vi "MoD Main-Optimize - Simulate.vi"() -> ()   [LabVIEW 2015]
uses:
  <vilib>/ni845x/ni845x.llb/ni845xControl.ctl
  <vilib>/addons/control/pid/pid.llb/PID Control Input Filter (DBL).vi
  <vilib>/addons/control/pid/autopid.llb/PID Online Autotuning (Relay Feedback).vi
  <vilib>/addons/control/pid/NI_PID_autopid.lvlib
  <vilib>/addons/control/pid/NI_PID_pid.lvlib
  <vilib>/DAQmx/read.llb/DAQmx Read (Analog 1D DBL NChan 1Samp).vi
  <vilib>/DAQmx/create/channels.llb/DAQmx Create Channel (AI-Voltage-Basic).vi
panel:
  out "stop_xl_write":bool=TRUE
  out "Num_exp_till_pause":i32
  out "Syringe_pump?":bool=TRUE
  out "System Error":bool=TRUE
  out "error out":errorcluster
  out "MS task":refnum<k21>
  out "MS Array":dbl[](array[numeric]) format="%0.2f"
  out "Pump setpoint(ul/min) 6":dbl format="%#_13g"
  out "Pump setpoint(ul/min) 5":dbl format="%#_13g"
  out "Pump setpoint(ul/min) 4":dbl format="%#_13g"
  out "Pump setpoint(ul/min) 3":dbl format="%#_13g"
  out "Pump setpoint(ul/min) 2":dbl format="%#_13g"
  out "Pump setpoint(ul/min) 1":dbl format="%#_13g"
  out "Volume (ul) 5":dbl format="%#_13g"
  out "Volume (ul) 4":dbl format="%#_13g"
  out "Volume (ul) 3":dbl format="%#_13g"
  out "Volume (ul) 2":dbl format="%#_13g"
  out "Volume (ul) 1":dbl format="%#_13g"
  in  "tau 5":dbl format="%#_13g"
  out "tau 4":dbl format="%#_13g"
  out "tau 3":dbl format="%#_13g"
  out "tau 2":dbl format="%#_13g"
  out "tau 1":dbl format="%#_13g"
  out "Reactor Length":dbl format="%#_13g"
  out "Flowrate Sensor 2":dbl format="%#_13g"
  out "Flowrate Sensor 1":dbl format="%#_13g"
  out "Pressure 2":dbl format="%#_13g"
  out "Pressure 1":dbl format="%#_13g"
  out "Temperature Control 5":bool=TRUE
  out "Temperature Control 4":bool=TRUE
  out "Temperature Control 3":bool=TRUE
  out "Temperature Control 2":bool=TRUE
  out "Temperature Control 1":bool=TRUE
  out "Temperature SP 5":dbl format="%#_g'C"
  out "Temperature SP 4":dbl format="%#_g'C"
  out "Temperature SP 3":dbl format="%#_g'C"
  out "Temperature SP 2":dbl format="%#_g'C"
  out "Temperature SP 1":dbl format="%#_g'C"
  in  "Bay Temperature 5":dbl
  in  "SSR Duration 5":dbl
  in  "SSR Duration 4":dbl
  in  "SSR Duration 3":dbl
  in  "SSR Duration 2":dbl
  in  "SSR Duration 1":dbl
  in  "Total Product Amount":dbl=1.0 format="%#_gml"
  out "Setup Error":bool=TRUE
  out "Error Message":string
  out "ID CTR":i32
  in  "Tab Control 2":enum32{"Faults", "Devices"}(tab)=enum."Devices"
  out "Fault Cluster":T1
  in  "COMM Port:: Harvard Syringe Pump":refnum<visa-resource-name>
  in  "Sample Valve COMM::Port":refnum<visa-resource-name>
  in  "Arduino COMM Port":refnum<visa-resource-name>
  in  "COMM Port :: Milligat Pumps":refnum<visa-resource-name>
  in  "IR Sensor Device":T2
  in  "MS Analog Channel":tag
  in  "Tab Control":T3(tab)
  in  "System decide help Button":bool
  in  "Reaction Scheme Confirm":bool
  in  "Synthesis Route Array":string[](array[string])=["Aldehyde", "Amine", "BoroHydride", "Aqueous Salt", "", ""]
  in  "Manual/Automated":bool
  in  "Save Button":bool
  in  "Open Button":bool
  in  "New rxn scheme button":bool
  in  "System decide help Button 2":bool
  out "Setup Confirm":bool=TRUE
  in  "BAY 1":u16(ring) items=["                 Bypass", "             Hot Reactor", "               Separator"]
  in  "BAY 5":u16(ring)=2 items=["                     Bypass", "                Hot Reactor", "                 Separator"]
  in  "BAY 4":u16(ring) items=["                     Bypass", "                Hot Reactor", "                  Separator"]
  in  "BAY 3":u16(ring)=1 items=["                     Bypass", "                 Hot Reactor", "                  Separator"]
  in  "BAY 2":u16(ring)=1 items=["                     Bypass", "                Hot Reactor", "                  Separator"]
  out "Paramter Confirm":bool=TRUE
  in  "System Parameters Help Button":bool
  in  "System Parameters Confirm Button":bool
  in  "Bay Parameters":T4={"Pump 1 Reagent Concentration"=2.0, "Pump 2 Reagent Concentration"=2.0, "Pump 3 Reagent Concentration"=2.0, "Pump 4 Reagent Concentration"=2.0, "Pump 5 Reagent Concentration"=2.0, "Bay 1 Parameters"={"Pump 1 Flowrate"=0.0, "optimize_temp"=TRUE, "optimize_tau"=TRUE, "Run at set flowrate"=FALSE, "Pump 2 Flowrate"=0.0, "Temperature Params"=[0.0, 25.0, 100.0], "Resisdence time params"=[0.0, 0.5, 15.0], "Resisdence time params 2"=[0.0, 0.5, 15.0]}, "Bay 2 Parameters"={"Pump 3 Flowrate"=0.0, "optimize_temp"=TRUE, "optimize_tau"=TRUE, "Run at set flowrate"=FALSE, "Temperature Params"=[0.0, 25.0, 100.0], "Resisdence time params"=[0.0, 0.5, 15.0], "pump_at_ratio"=FALSE, "pump_num_ratio"=0.0}, "Bay 3 Parameters"={"Pump 4 Flowrate"=0.0, "optimize_temp"=FALSE, "optimize_tau"=FALSE, "Run at set flowrate"=FALSE, "Temperature Params"=[0.0, 0.0, 0.0], "Resisdence time params"=[0.0, 0.0, 0.0], "pump_at_ratio"=TRUE, "pump_num_ratio"=1.5}, "Bay 4 Parameters"={"Pump 5 Flowrate"=0.0, "Run at set flowrate"=FALSE, "optimize_temp"=FALSE, "optimize_tau"=FALSE, "Resisdence time params"=[0.0, 0.0, 0.0], "Temperature Params"=[0.0, 0.0, 0.0], "pump_at_ratio"=FALSE, "pump_num_ratio"=0.0}, "Bay 5 Parameters"={"Pump 6 Flowrate"=0.0, "Run at set flowrate"=FALSE, "optimize_temp"=FALSE, "optimize_tau"=FALSE, "Resisdence time params"=[0.0, 0.0, 0.0], "Temperature Params"=[0.0, 0.0, 0.0], "pump_at_ratio"=FALSE, "pump_num_ratio"=0.0}, "Bay 1 Flow Rate Ratio \n(Pump 1: Pump 2)"=1.0, "tube_id(in)"=[enum.".03", enum.".03", enum.".03", enum.".03", enum.".03"], "xml_filename"="temp_xml", "Excel File Name"="C:\\Users\\HPLC\\Dropbox (MIT)\\MoD Files\\Data\\HWE Results\\HWE Optimization HPLC - 04112017 sim", "HPLC File Name"="C:\\Chem32\\1\\Data\\MOD", "Matlab File"="C:\\Users\\HPLC\\Dropbox (MIT)\\MoD Files\\Data\\04112017", "Syringe for Pump 2?"=TRUE, "Num_conditons_per_wait"=0.0, "Continue from previous optimization?"=FALSE, "Pump 6 Reagent Concentration"=2.0} {"Pump 6 Reagent Concentration" format="%#_6gM"; "Bay 5 Parameters"."Temperature Params" format="%#_g'C"; "Bay 4 Parameters"."Temperature Params" format="%#_g'C"; "Bay 3 Parameters"."Temperature Params" format="%#_g'C"; "Bay 2 Parameters"."Temperature Params" format="%#_g'C"; "Bay 1 Parameters"."Temperature Params" format="%#_g'C"; "Pump 5 Reagent Concentration" format="%#_6gM"; "Pump 4 Reagent Concentration" format="%#_6gM"; "Pump 3 Reagent Concentration" format="%#_6gM"; "Pump 2 Reagent Concentration" format="%#_6gM"; "Pump 1 Reagent Concentration" format="%#_6gM"}
  out "System Confirm Not Clicked":string
  in  "Debug_run_button":bool
  in  "Pump 1":bool
  in  "Flowrate 1":dbl=200.0
  in  "Pump 4":bool
  in  "Flowrate 4":dbl=200.0
  in  "Pump 5":bool
  in  "Flowrate 5":dbl=200.0
  in  "Pump 2":bool
  in  "Flowrate 2":dbl=200.0
  in  "Pump 3":bool
  in  "Flowrate 3":dbl=200.0
  in  "Pump 6":bool
  in  "Flowrate 6":dbl=200.0
  in  "Bay Heating 1":bool
  in  "Bay Heating 2":bool
  in  "Bay Heating 3":bool
  in  "Bay Heating 4":bool
  in  "Bay Heating 5":bool
  out "HPLC Analysis":bool
  out "Equlibrating Temperature":bool
  out "Flushing System":bool
  out "Calculate condition":bool
  out "System Flush Wait Time":u8(slide) scale=0.0..2150.711842843066
  out "Temperature 5":dbl format="%#_g'C"
  out "Temperature 4":dbl format="%#_g'C"
  out "Temperature 3":dbl format="%#_g'C"
  out "Temperature 2":dbl format="%#_g'C"
  out "Temperature 1":dbl format="%#_g'C"
  out "Flowrate Chart":T5(graph)
  out "Bay 5":u16(ring) items=["                     Bypass", "                   Reactor1", "               Separator"]
  out "Bay 4":u16(ring) items=["                     Bypass", "                   Reactor1", "               Separator"]
  out "Bay 3":u16(ring) items=["                     Bypass", "                   Reactor1", "               Separator"]
  out "Bay 2":u16(ring) items=["                     Bypass", "                   Reactor1", "               Separator"]
  out "Bay 1":u16(ring) items=["                     Bypass", "                   Reactor1", "               Separator"]
  out "Teperature Chart":T5(graph)
  out "Pump Setpoints Chart":T5(graph)
  out "Pressure Chart":T5(graph)
  out "MS Signals Chart":dbl[][](graph)
  out "Optimization_loop_index":i32
  out "curr_wait_time(min)":dbl
  out "total_flush_time(min)":dbl
  out "Temp SS? 5":bool=TRUE
  out "Temp SS? 4":bool=TRUE
  out "Temp SS? 3":bool=TRUE
  out "Temp SS? 2":bool=TRUE
  out "Temp SS? 1":bool=TRUE
  out "System Flushed?":bool
  out "stop_button clicked":bool
  out "Total System Resisdence Time(min)":dbl
  out "Stop":bool=TRUE
  in  "Run_Stop_cluster":T6
  # "Molecules on Demand"
  # "Synthesis Route"
  # "Reagent List"
  # "1"
  # "2"
  # "1"
  # "3"
  # "2"
  # "4"
  # "3"
  # "5"
  # "4"
  # "6"
  # "5"
  # "Product"
  # "6"
  # "Have system decide based on synthesis route"
  # "Manually enter bay configuration"
  # "System Schematic"
  # "Optimization Parameters"
  # "Bay"
  # "Tube ID (in)"
  # "1."
  # "2."
  # "3."
  # "4."
  # "5."
  # "Pause After Every"
  # "Experiments"
  # "Reporting"
  # "XML Output File Name"
  # "Excel Output File Name"
  # "HPLC File Path"
  # "MATLAB File Path"
  # "Temperature"
  # "Residence time(min)"
  # "Setpoint"
  # "Lower Bound"
  # "Upper Bound"
  # "Optimize?"
  # "-or-"
  # "Run at"
  # "times incoming flow"
  # "Temperature"
  # "Residence time(min)"
  # "Setpoint"
  # "Lower Bound"
  # "Upper Bound"
  # "Optimize?"
  # "-or-"
  # "Run at"
  # "times incoming flow"
  # "Temperature"
  # "Residence time(min)"
  # "Setpoint"
  # "Lower Bound"
  # "Upper Bound"
  # "Optimize?"
  # "-or-"
  # "Run at"
  # "times incoming flow"
  # "Temperature"
  # "Residence time(min)"
  # "Setpoint"
  # "Lower Bound"
  # "Upper Bound"
  # "Optimize?"
  # "-or-"
  # "Run at"
  # "times incoming flow"
  # "Temperature"
  # "Residence time(min)"
  # "Setpoint"
  # "Lower Bound"
  # "Upper Bound"
  # "Optimize?"
  # "Use this page to manually test the different functions of the system during standby mode"
  # "Pumps"
  # "Bay Heating"
  # "Temperature('C)"
  # "Pressure (psi)"
  # "Flowrate (ul/min)"
  # "Pump Flowrate Setpoints(ul/min)"
  # "MS Output Voltage"
  # "Experimental Steps"
  # "Calculated new conditions"
  # "Flushed System"
  # "Analyzed HPLC"
  # "Equilibrated Temperature"
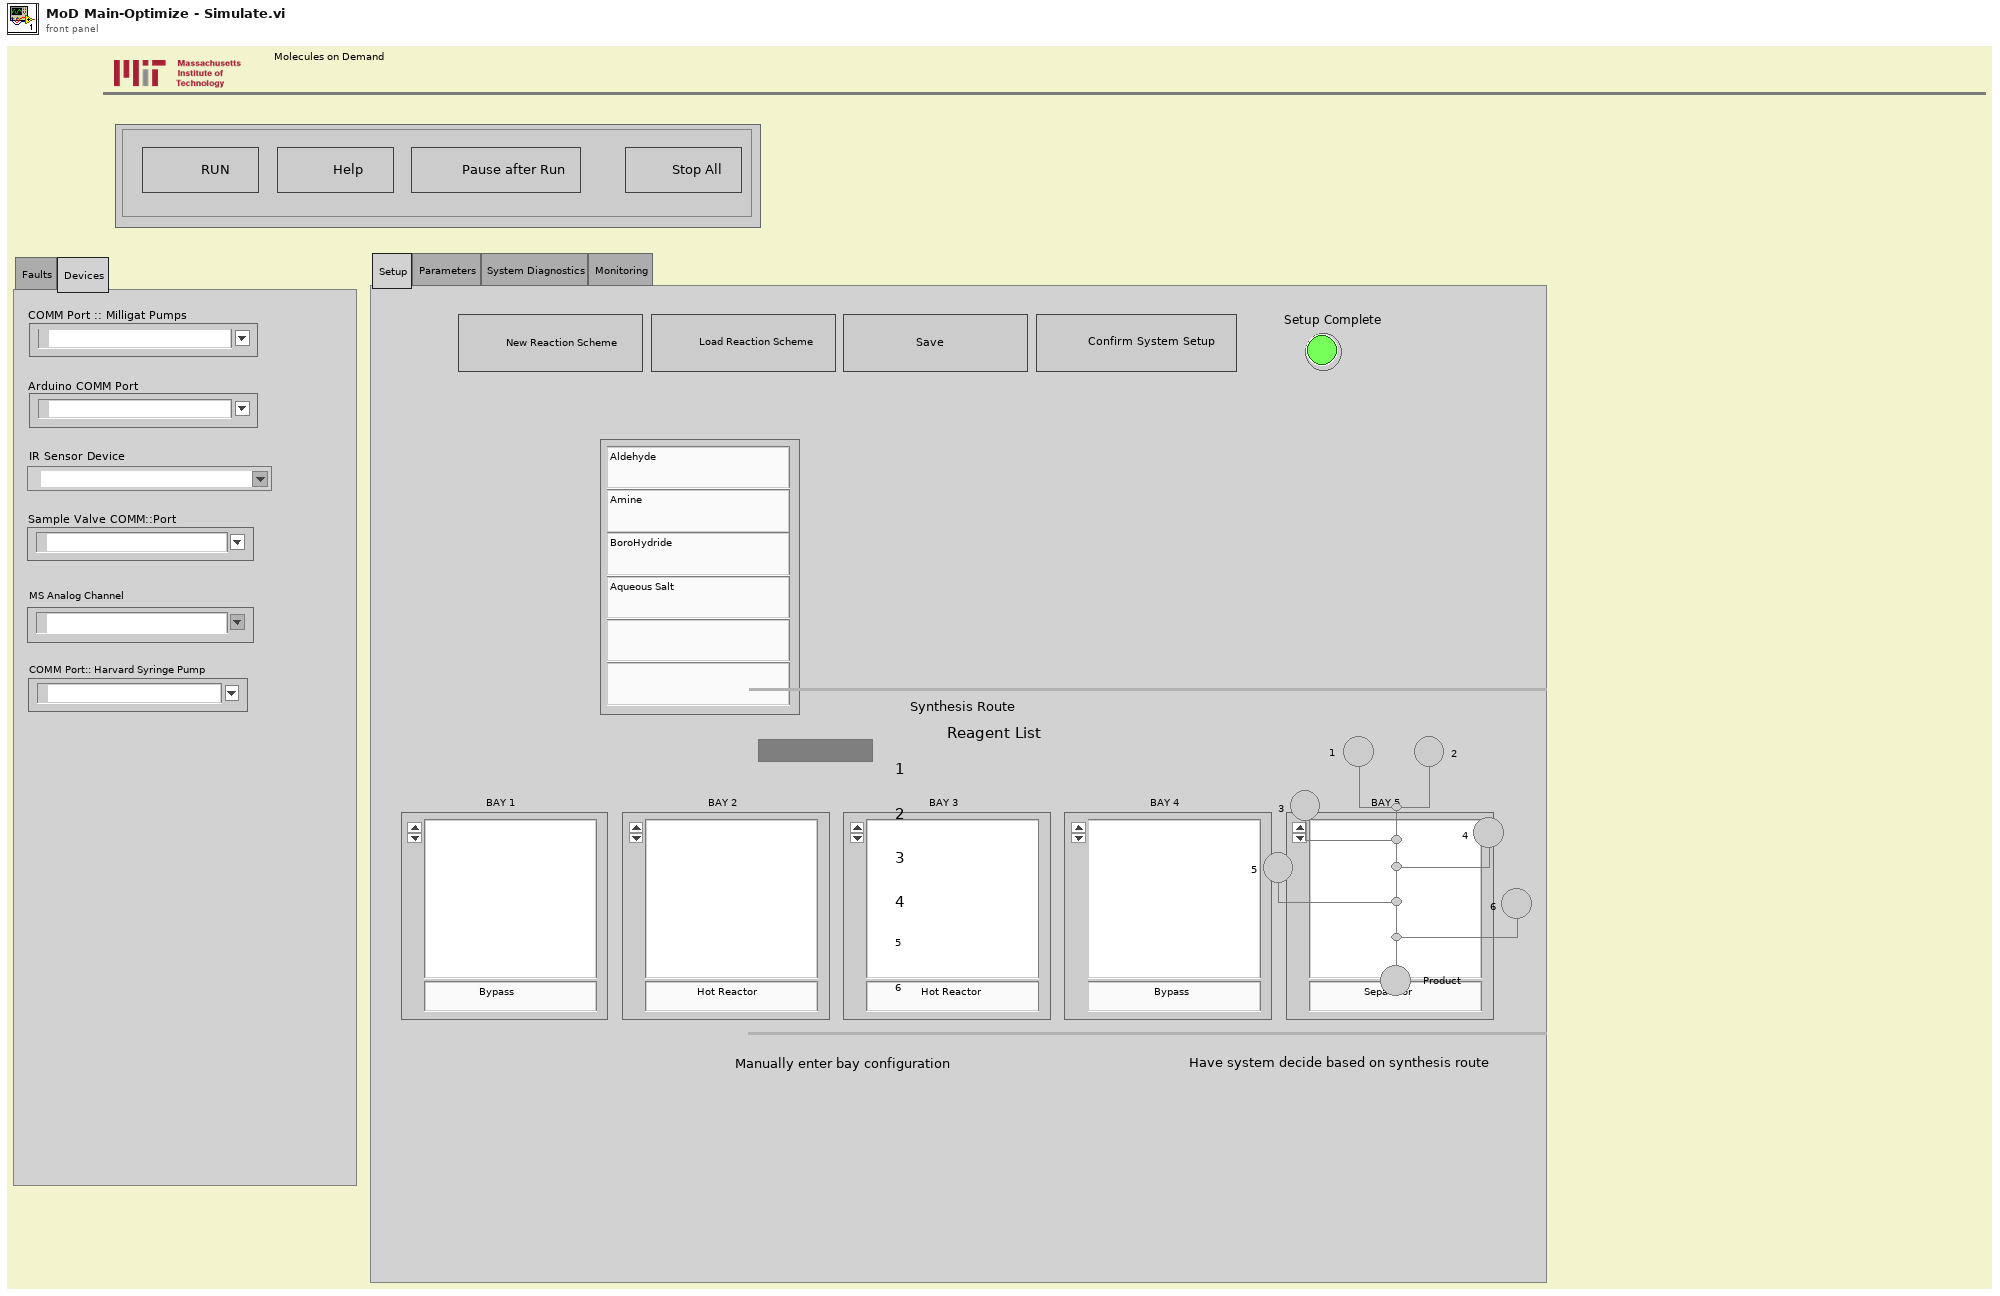
[diagram p1: front panel]
types:
  T1 = cluster{"Pump COMM Port":bool, "Pressure":bool, "Flow Rate":bool, "Temperature Sensor COMM Port":bool, "Arduino COMM Port":bool, "Chiller COMM Port":bool}
  T2 = typedef "ni845xControl.ctl" = refnum<k21>
  T3 = enum32{"Setup", "Parameters", "System Diagnostics", "Monitoring"}
  T4 = cluster{"Pump 1 Reagent Concentration":dbl, "Pump 2 Reagent Concentration":dbl, "Pump 3 Reagent Concentration":dbl, "Pump 4 Reagent Concentration":dbl, "Pump 5 Reagent Concentration":dbl, "Bay 1 Parameters":cluster{"Pump 1 Flowrate":dbl, "optimize_temp":bool, "optimize_tau":bool, "Run at set flowrate":bool, "Pump 2 Flowrate":dbl, "Temperature Params":dbl[], "Resisdence time params":dbl[], "Resisdence time params 2":dbl[]}, "Bay 2 Parameters":cluster{"Pump 3 Flowrate":dbl, "optimize_temp":bool, "optimize_tau":bool, "Run at set flowrate":bool, "Temperature Params":dbl[], "Resisdence time params":dbl[], "pump_at_ratio":bool, "pump_num_ratio":dbl}, "Bay 3 Parameters":cluster{"Pump 4 Flowrate":dbl, "optimize_temp":bool, "optimize_tau":bool, "Run at set flowrate":bool, "Temperature Params":dbl[], "Resisdence time params":dbl[], "pump_at_ratio":bool, "pump_num_ratio":dbl}, "Bay 4 Parameters":cluster{"Pump 5 Flowrate":dbl, "Run at set flowrate":bool, "optimize_temp":bool, "optimize_tau":bool, "Resisdence time params":dbl[], "Temperature Params":dbl[], "pump_at_ratio":bool, "pump_num_ratio":dbl}, "Bay 5 Parameters":cluster{"Pump 6 Flowrate":dbl, "Run at set flowrate":bool, "optimize_temp":bool, "optimize_tau":bool, "Resisdence time params":dbl[], "Temperature Params":dbl[], "pump_at_ratio":bool, "pump_num_ratio":dbl}, "Bay 1 Flow Rate Ratio \n(Pump 1: Pump 2)":dbl, "tube_id(in)":enum16{".01", ".02", ".03", ".04"}[], "xml_filename":string, "Excel File Name":string, "HPLC File Name":string, "Matlab File":string, "Syringe for Pump 2?":bool, "Num_conditons_per_wait":dbl, "Continue from previous optimization?":bool, "Pump 6 Reagent Concentration":dbl}
  T5 = cluster{"[0]":dbl, "[1]":dbl, "[2]":dbl, "[3]":dbl, "[4]":dbl, "[5]":dbl, "[6]":dbl, "[7]":dbl, "[8]":dbl}
  T6 = cluster{"Stop":bool, "Help Button":bool, "Run":bool, "Stop Run Button":bool}
  T7 = cluster{"Proportional gain Kc":dbl, "Integral time Ti (sec)":dbl, "Derivative time Ti (sec)":dbl}
  T8 = cluster{"type of controller":enum16{"P", "PI", "PID"}, "relay cycles":i32, "relay amplitude":dbl, "control specifications":enum16{"Fast", "Normal", "Slow"}, "PV noise level":dbl}
  T9 = cluster{"proportional gain (Kc)":dbl, "integral time (Ti, min)":dbl, "derivative time (Td, min)":dbl}
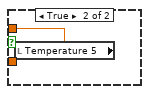
[diagram p6: hidden frame]
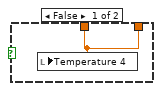
[diagram p7: hidden frame]
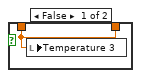
[diagram p8: hidden frame]
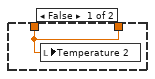
[diagram p9: hidden frame]
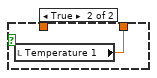
[diagram p10: hidden frame]
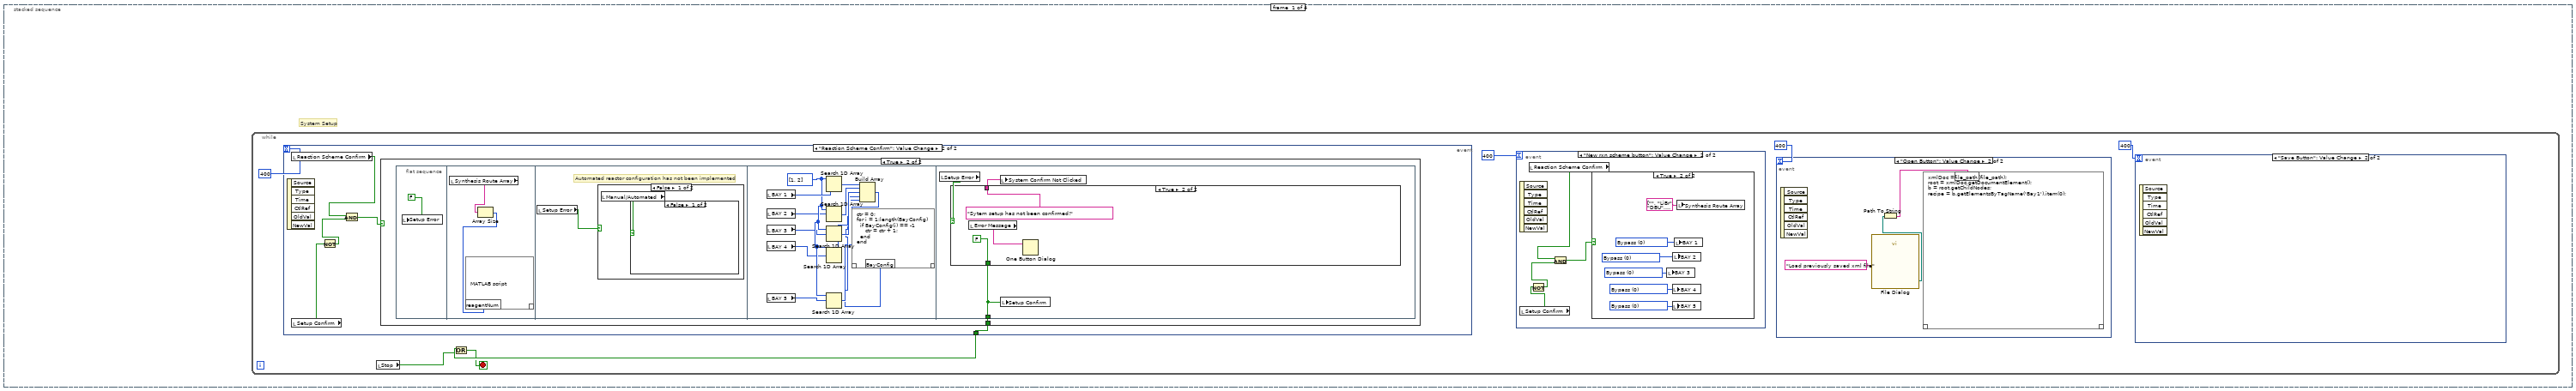
[diagram p11: hidden frame]
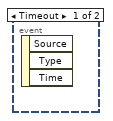
[diagram p12: hidden frame]
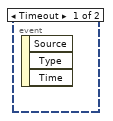
[diagram p13: hidden frame]
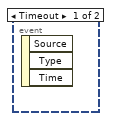
[diagram p14: hidden frame]
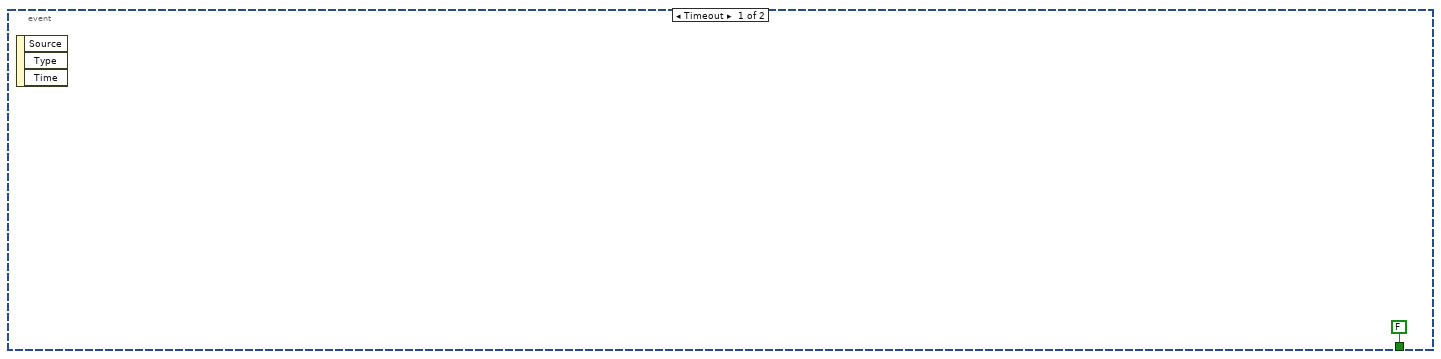
[diagram p16: hidden frame]
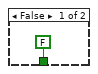
[diagram p17: hidden frame]
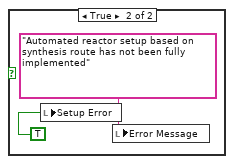
[diagram p18: hidden frame]
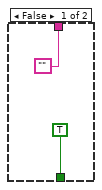
[diagram p20: hidden frame]
diagram:
  # "Assume User always uses the first bay first"
  n1 = flat-sequence {
    tunnel: ["COMM Port :: Milligat Pumps"] -> w3
    tunnel: ["Bay Parameters"] -> w1
    tunnel: [w37] -> w4
    tunnel: w3 -> [w37]
    tunnel: [w20] -> w2
    tunnel: w1 -> [w17]
    tunnel: w4 -> [w42]
    tunnel: w2 -> [w41]
    frame #0 {
      w7 = FALSE ("Equlibrating Temperature")
      "Stop" <- FALSE ("Stop")
      "ID CTR" <- 0
      "Setup Confirm" <- FALSE ("Setup Confirm")
      "Setup Error" <- FALSE ("Setup Error")
      "Reactor Length" <- 10.5
      "System Error" <- FALSE ("System Error")
      "Num_exp_till_pause" <- 0 ("Num_exp_till_pause")
      "Equlibrating Temperature" <- w7
      "Calculate condition" <- w7
      "Flushing System" <- w7
      "HPLC Analysis" <- w7
      "Paramter Confirm" <- FALSE ("Paramter Confirm")
      "stop_xl_write" <- FALSE ("stop_xl_write")
    }
    frame #1 {
      w31 = 23
      (unwired) path "C:/Users/User1/Documents/Lab/MoD/Images"
      n2 = disable-structure shown="Disabled" {
        frame Disabled {
          n3 = call-poly <vilib>:"DAQmx Create Virtual Channel.vi"("physical channels"="MS Analog Channel") -> ("task out"=→"MS task":refnum<k21>)  [unwired: 13 in, 1 out]
        }
        frame Enabled {
        }
      }
      n4 = local write "Debug_run_button"(TRUE) -> ()
      n5 = local read "BAY 2"() -> (w35:u16)
      n6 = local read "BAY 3"() -> (w34:u16)
      n7 = local read "BAY 4"() -> (w33:u16)
      n8 = local read "BAY 5"() -> (w32:u16)
      n9 = local read "BAY 1"() -> (w36:u16)
      n10 = local write "Bay 1"(w36) -> ()
      n11 = local write "Bay 2"(w35) -> ()
      n12 = local write "Bay 3"(w34) -> ()
      n13 = local write "Bay 4"(w33) -> ()
      n14 = local write "BAY 5"(w32) -> ()
      n15 = Unbundle By Name(w17) -> ("Syringe for Pump 2?"=→"Syringe_pump?":bool)
      n16 = local write "Temperature 1"(w31) -> ()
      n17 = local write "Temperature 2"(w31) -> ()
      n18 = local write "Temperature 3"(w31) -> ()
      n19 = local write "Temperature 4"(w31) -> ()
      n20 = local write "Temperature 5"(w31) -> ()
      n21 = local write "Temperature SP 1"(w31) -> ()
      n22 = local write "Temperature SP 2"(w31) -> ()
      n23 = local write "Temperature SP 3"(w31) -> ()
      n24 = local write "Temperature SP 4"(w31) -> ()
      n25 = local write "Temperature SP 5"(w31) -> ()
      n26 = Current VI's Path() -> (path=w24:path)
      n27 = Strip Path(path=w24) -> (stripped path=w22:path)  [unwired: 1 out]
      n28 = Strip Path(path=w22) -> (stripped path=w21:path)  [unwired: 1 out]
      n29 = Build Path(base path=w21, name or relative path="MATLAB") -> (appended path=w20:path)
      "Pump setpoint(ul/min) 1" <- 0.0 ("Pump setpoint(ul/min) 1")
      "Pump setpoint(ul/min) 2" <- 0.0 ("Pump setpoint(ul/min) 2")
      "Pump setpoint(ul/min) 3" <- 0.0 ("Pump setpoint(ul/min) 3")
      "Pump setpoint(ul/min) 4" <- 0.0 ("Pump setpoint(ul/min) 4")
      "Pump setpoint(ul/min) 5" <- 0.0 ("Pump setpoint(ul/min) 5")
      "Pump setpoint(ul/min) 6" <- 0.0 ("Pump setpoint(ul/min) 6")
    }
    frame #2 {
      # "Main Help Dialog Popup"
      n30 = while {
        stop <- w846 stop-if-true
        n31 = event shown="[0] Timeout" {
          selector: _ -> [_ _ _ _ _ _]
          dyn-events: _ -> [_ _ _ _ _ _]
          timeout: 500 -> [_ _ _ _ _ _]
          event Timeout {
            n32 = event-data() -> ()  [unwired: 1 in, 3 out]
          }
          event "Run_Stop_cluster.Help Button": Value Change {
            n33 = local read "Run_Stop_cluster"() -> (w849:T6)
            n34 = event-data() -> ()  [unwired: 1 in, 4 out]
            n35 = Unbundle By Name(w849) -> ("Help Button"=w848:bool)
            n36 = case shown="True" w848 {
              frame False {
              }
              frame True {
                n37 = call "help.vi"() -> ()  [unwired: 11 in]
              }
            }
          }
          event "System decide help Button": Value Change {
            n38 = event-data() -> ()  [unwired: 1 in, 5 out]
            n39 = call "help_synthesis_man-auto_instructions.vi"() -> ()  [unwired: 12 in]
          }
          event "System Parameters Help Button": Value Change {
            n40 = event-data() -> ()  [unwired: 1 in, 5 out]
            n41 = call "help_parameters_setup.vi"() -> ()  [unwired: 12 in]
          }
          event "System decide help Button 2": Value Change {
            n42 = event-data() -> ()  [unwired: 1 in, 5 out]
            n43 = call "help_synthesis_route_instructions.vi"() -> ()  [unwired: 12 in]
          }
          event "Run_Stop_cluster.Stop": Value Change {
            n44 = event-data() -> ()  [unwired: 1 in, 5 out]
            n45 = local write "Stop"(TRUE) -> ()
          }
        }
        n46 = local read "Stop"() -> (w846:bool)
      }
      n47 = stacked-sequence {
        tunnel: w42 -> [_ _ _ _]
        tunnel: w41 -> [_ w201 _ _]
        frame #0 {
          # "System Setup"
          n48 = while {
            stop <- w147 stop-if-true
            n49 = event shown="[1] \"Reaction Scheme Confirm\": Value Change" {
              selector: _ -> [_ _]
              dyn-events: _ -> [_ _]
              timeout: 400 -> [_ _]
              tunnel: [FALSE w165] -> w149
              event Timeout {
                n50 = event-data() -> ()  [unwired: 1 in, 3 out]
              }
              event "Reaction Scheme Confirm": Value Change {
                n51 = event-data() -> ()  [unwired: 1 in, 6 out]
                n52 = local read "Reaction Scheme Confirm"() -> (w169:bool)
                n53 = local read "Setup Confirm"() -> (w167:bool)
                n54 = Not(x=w167) -> (.not. x?=w166:bool)
                n55 = And(x=w169, y=w166) -> (x .and. y?=w168:bool)
                n56 = case shown="True" w168 {
                  tunnel: [FALSE w171] -> w165
                  frame False {
                  }
                  frame True {
                    n57 = flat-sequence {
                      tunnel: [w191] -> w171
                      frame #0 {
                        n58 = local write "Setup Error"(FALSE) -> ()
                      }
                      frame #1 {
                        n59 = local read "Synthesis Route Array"() -> (w174:string[])
                        n60 = Array Size(array=w174) -> (size(s)=w173:i32)
                        n61 = script code="MATLAB script"("reagentNum"=w173) -> ()  [unwired: 1 in, 1 out]
                      }
                      frame #2 {
                        # "Automated reactor configuration has not been implemented"
                        n62 = local read "Setup Error"() -> (w175:bool)
                        n63 = case shown="False" w175 {
                          frame False {
                            n64 = local read "Manual/Automated"() -> (w176:bool)
                            n65 = case shown="False" w176 {
                              frame False {
                              }
                              frame True {
                                n66 = local write "Setup Error"(TRUE ("Setup Error")) -> ()
                                n67 = local write "Error Message"("Automated reactor setup based on synthesis route has not been fully implemented") -> ()
                              }
                            }
                          }
                          frame True {
                          }
                        }
                      }
                      frame #3 {
                        w189 = i32[] [1, 2]
                        n68 = local read "BAY 1"() -> (w190:u16)
                        n69 = local read "BAY 2"() -> (w188:u16)
                        n70 = local read "BAY 3"() -> (w187:u16)
                        n71 = local read "BAY 4"() -> (w186:u16)
                        n72 = local read "BAY 5"() -> (w185:u16)
                        n73 = Search 1D Array(1D array=w189, element=w190) -> (index of element=w184:i32)  [unwired: 1 in]
                        n74 = Search 1D Array(1D array=w189, element=w188) -> (index of element=w183:i32)  [unwired: 1 in]
                        n75 = Search 1D Array(1D array=w189, element=w187) -> (index of element=w182:i32)  [unwired: 1 in]
                        n76 = Search 1D Array(1D array=w189, element=w186) -> (index of element=w181:i32)  [unwired: 1 in]
                        n77 = Search 1D Array(1D array=w189, element=w185) -> (index of element=w180:i32)  [unwired: 1 in]
                        n78 = Build Array(w184, w183, w182, w181, w180) -> (w179:i32[])
                        n79 = script code="ctr = 0;\nfor i = 1:length(BayConfig)\n  if BayConfig(i) == -1\n     ctr = ctr + 1;\n  end\nend"("BayConfig"=w179) -> ()  [unwired: 1 in, 1 out]
                      }
                      frame #4 {
                        n80 = local read "Setup Error"() -> (w193:bool)
                        n81 = case shown="True" w193 {
                          tunnel: [TRUE FALSE] -> w191
                          tunnel: ["" "Sytem setup has not been confirmed!"] -> w192
                          frame False {
                          }
                          frame True {
                            n82 = local read "Error Message"() -> (w198:string)
                            n83 = One Button Dialog(message=w198) -> ()  [unwired: 1 in, 1 out]
                          }
                        }
                        n84 = local write "System Confirm Not Clicked"(w192) -> ()
                        n85 = local write "Setup Confirm"(w191) -> ()
                      }
                    }
                  }
                }
              }
            }
            n86 = local read "Stop"() -> (w148:bool)
            n87 = Or(x=w149, y=w148) -> (x .or. y?=w147:bool)
            n88 = event shown="[1] \"New rxn scheme button\": Value Change" {
              selector: _ -> [_ _]
              dyn-events: _ -> [_ _]
              timeout: 400 -> [_ _]
              event Timeout {
                n89 = event-data() -> ()  [unwired: 1 in, 3 out]
              }
              event "New rxn scheme button": Value Change {
                n90 = event-data() -> ()  [unwired: 1 in, 6 out]
                n91 = local read "Setup Confirm"() -> (w154:bool)
                n92 = local read "Reaction Scheme Confirm"() -> (w155:bool)
                n93 = Not(x=w154) -> (.not. x?=w157:bool)
                n94 = And(x=w155, y=w157) -> (x .and. y?=w156:bool)
                n95 = case shown="True" w156 {
                  frame False {
                  }
                  frame True {
                    w158 = u16 0 items=["                     Bypass", "                Hot Reactor", "                 Separator"] ("BAY 5")
                    w159 = u16 0 items=["                     Bypass", "                Hot Reactor", "                  Separator"] ("BAY 4")
                    w160 = u16 0 items=["                     Bypass", "                 Hot Reactor", "                  Separator"] ("BAY 3")
                    w161 = u16 0 items=["                     Bypass", "                Hot Reactor", "                  Separator"] ("BAY 2")
                    w162 = u16 0 items=["                 Bypass", "             Hot Reactor", "               Separator"] ("BAY 1")
                    n96 = local write "BAY 3"(w160) -> ()
                    n97 = local write "BAY 4"(w159) -> ()
                    n98 = local write "BAY 5"(w158) -> ()
                    n99 = local write "BAY 2"(w161) -> ()
                    n100 = local write "BAY 1"(w162) -> ()
                    n101 = local write "Synthesis Route Array"(string[] ["", "LiBr", "DBU", "Aldehyde", "Water", "Toluene"] ("Synthesis Route Array")) -> ()
                  }
                }
              }
            }
            n102 = event shown="[1] \"Open Button\": Value Change" {
              selector: _ -> [_ _]
              dyn-events: _ -> [_ _]
              timeout: 400 -> [_ _]
              event Timeout {
                n103 = event-data() -> ()  [unwired: 1 in, 3 out]
              }
              event "Open Button": Value Change {
                n104 = event-data() -> ()  [unwired: 1 in, 6 out]
                n105 = call "File Dialog"("prompt"="Load previously saved xml file") -> ("selected path"=w152:path)  [unwired: 11 in, 3 out]
                n106 = Path To String(path=w152) -> (string=w151:string)
                n107 = script code="xmlDoc = xmlread(file_path);\nroot = xmlDoc.getDocumentElement();\nb = root.getChildNodes;\nrecipe = b.getElementsByTagName('Bay1').item(0);"("file_path"=w151) -> ()  [unwired: 1 in, 1 out]
              }
            }
            n108 = event shown="[1] \"Save Button\": Value Change" {
              selector: _ -> [_ _]
              dyn-events: _ -> [_ _]
              timeout: 400 -> [_ _]
              event Timeout {
                n109 = event-data() -> ()  [unwired: 1 in, 3 out]
              }
              event "Save Button": Value Change {
                n110 = event-data() -> ()  [unwired: 1 in, 6 out]
              }
            }
          }
        }
        frame #1 {
          n111 = local read "Stop"() -> (w200:bool)
          n112 = Not(x=w200) -> (.not. x?=w199:bool)
          n113 = case shown="True" w199 {
            tunnel: w201 -> [_ w204]
            frame False {
              "stop_button clicked" <- TRUE ("stop_button clicked")
            }
            frame True {
              # "Parameters Initilization"
              n114 = flat-sequence {
                tunnel: [w214] -> w209
                tunnel: [w213] -> w208
                tunnel: [w212] -> w207
                tunnel: [w211] -> w206
                tunnel: [w210] -> w205
                tunnel: w209 -> [w226]
                tunnel: w208 -> [w225]
                tunnel: w207 -> [w224]
                tunnel: w206 -> [w223]
                tunnel: w205 -> [w222]
                tunnel: w204 -> [w216]
                tunnel: [w215] -> w203
                tunnel: w203 -> [w364]
                frame #0 {
                  # "Setup bays(RFID - verify)"
                  n115 = local read "BAY 1"() -> (w214:u16)
                  n116 = local read "BAY 2"() -> (w213:u16)
                  n117 = local read "BAY 3"() -> (w212:u16)
                  n118 = local read "BAY 4"() -> (w211:u16)
                  n119 = local read "BAY 5"() -> (w210:u16)
                  n120 = local write "Bay 1"(w214) -> ()
                  n121 = local write "Bay 2"(w213) -> ()
                  n122 = local write "Bay 3"(w212) -> ()
                  n123 = local write "Bay 4"(w211) -> ()
                  n124 = local write "Bay 5"(w210) -> ()
                }
                frame #1 {
                  n125 = while {
                    tunnel: w226 -> [w246]
                    tunnel: w225 -> [w245]
                    tunnel: w224 -> [w244]
                    tunnel: w223 -> [w243]
                    tunnel: w222 -> [w242]
                    tunnel: [w241] -> w221
                    tunnel: [w240] -> w220
                    tunnel: [w239] -> w219
                    tunnel: [w238] -> w218
                    tunnel: [w237] -> w217
                    tunnel: w216 -> [w228]
                    tunnel: [w227] -> w215
                    stop <- w236 stop-if-true
                    n126 = flat-sequence {
                      tunnel: w242 -> [w247]
                      tunnel: w243 -> [w248]
                      tunnel: w244 -> [w249]
                      tunnel: w245 -> [w250]
                      tunnel: w246 -> [w251]
                      tunnel: [w251] -> w233
                      tunnel: [w250] -> w232
                      tunnel: [w249] -> w231
                      tunnel: [w248] -> w230
                      tunnel: [w247] -> w229
                      tunnel: [w350] -> w241
                      tunnel: [w349] -> w240
                      tunnel: [w348] -> w239
                      tunnel: [w347] -> w238
                      tunnel: [w346] -> w237
                      tunnel: [w302] -> w227
                      tunnel: w233 -> [w362]
                      tunnel: w232 -> [w361]
                      tunnel: w231 -> [w360]
                      tunnel: w230 -> [w359]
                      tunnel: w229 -> [w358]
                      tunnel: w228 -> [w298]
                      frame #0 {
                        n127 = while {
                          stop <- w255 stop-if-true
                          n128 = event shown="[1] \"System Parameters Confirm Button\": Value Change" {
                            selector: _ -> [_ _]
                            dyn-events: _ -> [_ _]
                            timeout: u32 200 ("milliseconds to wait") -> [_ _]
                            tunnel: [FALSE TRUE] -> w253
                            event Timeout {
                              n129 = event-data() -> ()  [unwired: 1 in, 3 out]
                            }
                            event "System Parameters Confirm Button": Value Change {
                              n130 = event-data() -> ()  [unwired: 1 in, 5 out]
                              n131 = local write "System Parameters Confirm Button"(FALSE) -> ()
                            }
                          }
                          n132 = Wait (ms)(milliseconds to wait=u32 500) -> ()  [unwired: 1 out]
                          n133 = local read "Stop"() -> (w256:bool)
                          n134 = Or(x=w256, y=w253) -> (x .or. y?=w255:bool)
                        }
                      }
                      frame #1 {
                        # "Do while parameters have not been correctly entered"
                        n135 = local read "Bay Parameters"() -> (w261:T4)
                        n136 = local read "Synthesis Route Array"() -> (w275:string[])
                        n137 = Unbundle By Name(w261) -> ("Bay 1 Flow Rate Ratio \n(Pump 1: Pump 2)"=w301:dbl)
                        n138 = Unbundle By Name(w261) -> ("Continue from previous optimization?"=w297:bool)
                        n139 = Unbundle By Name(w261) -> ("Bay 1 Parameters.Run at set flowrate"=w345:bool)
                        n140 = Unbundle By Name(w261) -> ("Bay 1 Parameters.Pump 1 Flowrate"=w356:dbl)
                        n141 = Unbundle By Name(w261) -> ("Bay 1 Parameters.Pump 2 Flowrate"=w355:dbl)
                        n142 = Unbundle By Name(w261) -> ("Bay 2 Parameters.Run at set flowrate"=w343:bool)
                        n143 = Unbundle By Name(w261) -> ("Bay 2 Parameters.Pump 3 Flowrate"=w354:dbl)
                        n144 = Unbundle By Name(w261) -> ("Bay 3 Parameters.Pump 4 Flowrate"=w353:dbl)
                        n145 = Unbundle By Name(w261) -> ("Bay 3 Parameters.Run at set flowrate"=w342:bool)
                        n146 = Unbundle By Name(w261) -> ("Bay 4 Parameters.Run at set flowrate"=w339:bool)
                        n147 = Unbundle By Name(w261) -> ("Bay 4 Parameters.Pump 5 Flowrate"=w352:dbl)
                        n148 = Unbundle By Name(w261) -> ("Bay 5 Parameters.Pump 6 Flowrate"=w351:dbl)
                        n149 = Unbundle By Name(w261) -> ("Bay 5 Parameters.Run at set flowrate"=w338:bool)
                        n150 = Unbundle By Name(w261) -> ("Excel File Name"=w299:string)
                        n151 = Unbundle By Name(w261) -> ("Matlab File"=w295:string)
                        n152 = Unbundle By Name(w261) -> ("xml_filename"=w300:string)
                        n153 = Unbundle By Name(w261) -> ("Pump 3 Reagent Concentration"=w266:dbl)
                        n154 = Unbundle By Name(w261) -> ("Pump 2 Reagent Concentration"=w267:dbl)
                        n155 = Unbundle By Name(w261) -> ("Pump 4 Reagent Concentration"=w265:dbl)
                        n156 = Unbundle By Name(w261) -> ("Pump 5 Reagent Concentration"=w264:dbl)
                        n157 = Unbundle By Name(w261) -> ("Pump 6 Reagent Concentration"=w263:dbl)
                        n158 = Unbundle By Name(w261) -> ("Pump 1 Reagent Concentration"=w268:dbl)
                        n159 = Unbundle By Name(w261) -> ("tube_id(in)"=w357:enum16{".01", ".02", ".03", ".04"}[])
                        n160 = Index Array(array=w275, index=0) -> (element=w274:string)
                        n161 = Boolean To (0,1)(Boolean=w343) -> (0, 1=w294:i16)
                        n162 = Boolean To (0,1)(Boolean=w339) -> (0, 1=w340:i16)
                        n163 = Boolean To (0,1)(Boolean=w342) -> (0, 1=w341:i16)
                        n164 = Boolean To (0,1)(Boolean=w297) -> (0, 1=w296:i16)
                        n165 = Boolean To (0,1)(Boolean=w345) -> (0, 1=w344:i16)
                        n166 = Boolean To (0,1)(Boolean=w338) -> (0, 1=w337:i16)
                        n167 = Index Array(array=w275, index=1) -> (element=w269:string)
                        n168 = Build Array(w268, w267, w266, w265, w264, w263) -> (w262:dbl[])
                        n169 = Index Array(array=w275, index=2) -> (element=w270:string)
                        n170 = Unbundle By Name(w261) -> ("Bay 1 Parameters.optimize_temp"=w336:bool)
                        n171 = Unbundle By Name(w261) -> ("Bay 1 Parameters.optimize_tau"=w334:bool)
                        n172 = Unbundle By Name(w261) -> ("Bay 2 Parameters.optimize_temp"=w332:bool)
                        n173 = Unbundle By Name(w261) -> ("Bay 2 Parameters.optimize_tau"=w330:bool)
                        n174 = Unbundle By Name(w261) -> ("Bay 3 Parameters.optimize_temp"=w328:bool)
                        n175 = Unbundle By Name(w261) -> ("Bay 3 Parameters.optimize_tau"=w326:bool)
                        n176 = Unbundle By Name(w261) -> ("Bay 4 Parameters.optimize_temp"=w324:bool)
                        n177 = Unbundle By Name(w261) -> ("Bay 4 Parameters.optimize_tau"=w322:bool)
                        n178 = Index Array(array=w275, index=3) -> (element=w271:string)
                        n179 = Boolean To (0,1)(Boolean=w324) -> (0, 1=w323:i16)
                        n180 = Boolean To (0,1)(Boolean=w322) -> (0, 1=w321:i16)
                        n181 = Index Array(array=w275, index=4) -> (element=w272:string)
                        n182 = Boolean To (0,1)(Boolean=w326) -> (0, 1=w325:i16)
                        n183 = Boolean To (0,1)(Boolean=w332) -> (0, 1=w331:i16)
                        n184 = Boolean To (0,1)(Boolean=w336) -> (0, 1=w335:i16)
                        n185 = Boolean To (0,1)(Boolean=w330) -> (0, 1=w329:i16)
                        n186 = Boolean To (0,1)(Boolean=w334) -> (0, 1=w333:i16)
                        n187 = Boolean To (0,1)(Boolean=w328) -> (0, 1=w327:i16)
                        n188 = Unbundle By Name(w261) -> ("Bay 5 Parameters.optimize_temp"=w320:bool)
                        n189 = Unbundle By Name(w261) -> ("Bay 5 Parameters.optimize_tau"=w318:bool)
                        n190 = Index Array(array=w275, index=5) -> (element=w273:string)
                        n191 = Boolean To (0,1)(Boolean=w320) -> (0, 1=w319:i16)
                        n192 = Boolean To (0,1)(Boolean=w318) -> (0, 1=w317:i16)
                        n193 = Build Array(w335, w333, w331, w329, w327, w325, w323, w321, w319, w317) -> (w316:i16[])
                        n194 = Unbundle By Name(w261) -> ("Bay 1 Parameters.Temperature Params"=w313:dbl[])
                        n195 = Unbundle By Name(w261) -> ("Bay 1 Parameters.Resisdence time params"=w308:dbl[])
                        n196 = Unbundle By Name(w261) -> ("Bay 2 Parameters.Temperature Params"=w312:dbl[])
                        n197 = Unbundle By Name(w261) -> ("Bay 2 Parameters.Resisdence time params"=w307:dbl[])
                        n198 = Unbundle By Name(w261) -> ("Bay 3 Parameters.Temperature Params"=w311:dbl[])
                        n199 = Unbundle By Name(w261) -> ("Bay 3 Parameters.Resisdence time params"=w306:dbl[])
                        n200 = Unbundle By Name(w261) -> ("Bay 4 Parameters.Temperature Params"=w310:dbl[])
                        n201 = Unbundle By Name(w261) -> ("Bay 4 Parameters.Resisdence time params"=w305:dbl[])
                        n202 = Unbundle By Name(w261) -> ("Bay 5 Parameters.Temperature Params"=w309:dbl[])
                        n203 = Unbundle By Name(w261) -> ("Bay 5 Parameters.Resisdence time params"=w304:dbl[])
                        n204 = Unbundle By Name(w261) -> ("Bay 1 Parameters.Resisdence time params 2"=w260:dbl[])
                        n205 = Unbundle By Name(w261) -> ("Bay 3 Parameters.pump_num_ratio"=w288:dbl)
                        n206 = Unbundle By Name(w261) -> ("Bay 4 Parameters.pump_num_ratio"=w285:dbl)
                        n207 = Unbundle By Name(w261) -> ("Bay 5 Parameters.pump_num_ratio"=w282:dbl)
                        n208 = Unbundle By Name(w261) -> ("Bay 2 Parameters.pump_num_ratio"=w291:dbl)
                        n209 = Unbundle By Name(w261) -> ("Bay 4 Parameters.pump_at_ratio"=w287:bool)
                        n210 = Boolean To (0,1)(Boolean=w287) -> (0, 1=w286:i16)
                        n211 = Unbundle By Name(w261) -> ("Bay 3 Parameters.pump_at_ratio"=w290:bool)
                        n212 = Boolean To (0,1)(Boolean=w290) -> (0, 1=w289:i16)
                        n213 = Unbundle By Name(w261) -> ("Bay 5 Parameters.pump_at_ratio"=w284:bool)
                        n214 = Boolean To (0,1)(Boolean=w284) -> (0, 1=w283:i16)
                        n215 = Unbundle By Name(w261) -> ("Bay 2 Parameters.pump_at_ratio"=w293:bool)
                        n216 = Boolean To (0,1)(Boolean=w293) -> (0, 1=w292:i16)
                        n217 = script code="length_reactor1 = 188;%cm\nsystem_error = 0;\nlength_reactor2 = 99; %cm\nlength_bypass = 10;%cm\nnumPeaks = 1;\nstart_phase_time = 1;\nFvalues = [];\nHPLC_Area = [];\ntube_diameters = [.01, .02, .03, .04];\nD1 = tube_diameters(tube_id(1) +1); D1 = D1*2.54;\nD2 = tube_diameters(tube_id(2) +1); D2 = D2*2.54;\nD3 = tube_diameters(tube_id(3) +1); D3 = D3*2.54;\nD4 = tube_diameters(tube_id(4) +1); D4 = D4*2.54;\nD5 = tube_diameters(tube_id(5) +1); D5 = D5*2.54;\nT1_span = [1 1]; T2_span = [1 1]; T3_span = [1 1]; T4_span = [1 1]; T5_span = [1 1];\n p1_span =  [1 1]; p2_span =  [1 1]; p3_span =  [1 1]; p4_span =  [1 1]; p5_span =  [1 1];  p6_span =  [1 1];\nOpt_params = [0 0 0 0 0 0 0 0 0 0 0];\nopt_ctr = 0;ncall = 100;\nrecord_data = true;\nT1_SP = 23; T2_SP = 23; T3_SP = 23; T4_SP = 23; T5_SP = 23;\nno_errors = 1;\nP1 = 0; P2 =0; P3 = 0; P4 = 0; P5 = 0; P6 = 0;\nis_first_set_of_exp = true;\nerror_message = 'System has no errors to report';\n%addpath(genpath('C:\\Users\\HPLC\\Dropbox (MIT)\\multistep_optimization'))\naddpath(genpath('C:\\Users\\HPLC\\Dropbox (MIT)\\MoD Files\\MATLAB'))\nallMSData = [];\nallHPLCData = [];\nallHPLCFile = [];\nCurrExp = 1;\nif Continue\n   load(matlabsavefile);\nelse\nx = []\n   IRSteadystate = 0;\n   ProductVec = [];\n   TwopointbaselineProductVec=[];\nend\nall_MSData = [];\n% ****************************************************************************************************\nif Bay1 == 1\n    %1.05m reactor\n     Vr1 = length_reactor1*D1^2/4*3.14159*1000;\n     if  Optimize_params(1)\n       % if choice is made to optimize temperature\n        if T1_params(2) < T1_params(3)\n             T1_span = [T1_params(2) ,  T1_params(3)];\n              Opt_params(1) = 1;\n         else\n            no_errors = 0;\n            error_message = 'Lower bound of temperature must be lower than upper bound';\n        end\n    else\n       %  if choice is made to not optimize temperature\n        T1_SP = T1_params(1);  \n    end\n\n    if Optimize_params(2)\n       % if user wants to optimize flowrates\n        if pump1_params(2) < pump1_params(3)\n             p1_span = [pump1_params(2) ,  pump1_params(3)];\n             p1_span = p1_span;\n             Opt_params(6) = 1; Opt_params(7) = 1;\n         else\n            no_errors = 0;\n            error_message = 'Lower bound of flowrate 1 must be lower than upper bound';\n        end\n         if pump2_params(2) < pump2_params(3)\n             p2_span = [pump2_params(2) ,  pump2_params(3)];\n             p2_span = p2_span;\n             Opt_params(6) = 1; Opt_params(7) = 1;\n         else\n            no_errors = 0;\n            error_message = 'Lower bound of flowrate 2 must be lower than upper bound';\n        end \n    else\n       if use_flowrate1\n            if P1_setrate < 0 || P2_setrate < 0\n               no_errors = 0;\n               error_message = 'Pump set flowrates can not be negative';\n            else\n               P1 = P1_setrate;\n               P2 = P1_setrate;\n            end\n       else\n            if pump1_params(1) > 0\n               P1 = pump1_params(1);\n            elseif not(isempty(pump1_chem))\n               no_errors = 0;\n               error_message = 'Bay1 Pump 1 setpoint must be greater than zero';\n            end\n             if pump2_params(1) > 0\n               P2 = pump2_params(1);\n            elseif not(isempty(pump2_chem))\n               no_errors = 0;\n               error_message = 'Bay1 Pump 2 setpoint must be greater than zero';\n            end\n       end\n    end\nelseif Bay1 == 0\n    % .1m bypass\n    Vr1 =length_bypass*D1^2/4*3.14159*1000;\n    if Optimize_params(1)\n          no_errors = 0;\n          error_message = 'Can not optimize temperature on bypass ';\n    end\n\n    if Optimize_params(2)\n       % if user wants to optimize residence time\n        if pump1_params(2) < pump1_params(3)\n             p1_span = [pump1_params(2) ,  pump1_params(3)];\n             p1_span = p1_span;\n             Opt_params(6) = 1; Opt_params(7) = 1;\n         else\n            no_errors = 0;\n            error_message = 'Lower bound of pump 1 must be lower than upper bound';\n        end\n       if pump2_params(2) < pump2_params(3)\n             p2_span = [pump2_params(2) ,  pump2_params(3)];\n             p2_span = p2_span;\n             Opt_params(6) = 1; Opt_params(7) = 1;\n         else\n            no_errors = 0;\n            error_message = 'Lower bound of pump 2 must be lower than upper bound';\n        end\n    else\n       if use_flowrate1\n            if P1_setrate < 0 || P2_setrate < 0\n               no_errors = 0;\n               error_message = 'Pump set flowrates can not be negative';\n            else\n               P1 = P1_setrate;\n               P2 = P2_setrate;\n            end\n       else\n            if pump1_params(1) > 0\n               P1 = pump1_params(1);\n            elseif not(isempty(pump1_chem))\n               no_errors = 0;\n               error_message = 'Bay 1 Pump 2 setpoint must be greater than zero';\n            end\n           if pump2_params(1) > 0\n               P2 = pump2_params(1);\n            elseif not(isempty(pump2_chem))\n               no_errors = 0;\n               error_message = 'Bay 1 Pump 2 setpoint must be greater than zero';\n            end\n       end\n    end\nelse\n    %separator\n    Vr1 = 1000;\n    if use_flowrate1\n        P1 = P1_setrate;\n        P2 = P2_setrate;\n    else \n        if not(isempty(pump1_chem))\n           P1 = 200;\n        end\n        if not(isempty(pump2_chem))\n           P2 = 200;\n        end\n    end\n    \nend\n\n% ****************************************************************************************************\n\n   if Bay2 == 1 \n   %1.05m reactor\n     Vr2 =length_reactor1*D2^2/4*3.14159*1000;\n     if  Optimize_params(3)\n       % if choice is made to optimize temperature\n        if T2_params(2) < T2_params(3)\n             T2_span = [T2_params(2) ,  T2_params(3)];\n             Opt_params(2) = 1;\n         else\n            no_errors = 0;\n            error_message = 'Lower bound of temperature must be lower than upper bound';\n        end\n    else\n       %  if choice is made to not optimize temperature\n        T2_SP = T2_params(1);  \n    end\n\n    if Optimize_params(4)\n       % if user wants to optimize residence time\n        if pump3_params(2) < pump3_params(3)\n             p3_span = [pump3_params(2) ,  pump3_params(3)];\n             p3_span = p3_span;\n             Opt_params(8) = 1;\n         else\n            no_errors = 0;\n            error_message = 'Lower bound of pump 3 must be lower than upper bound';\n        end\n    else\n       if use_flowrate2\n            if P3_setrate < 0\n               no_errors = 0;\n               error_message = 'Pump set flowrates can not be negative';\n            else\n               P3 = P3_setrate;\n            end\n       elseif Bay2_ratio\n            P3 = Bay2_pump_ratio*(P1); % changed from Bay2_pump_ratio*(P1+P2); \n       else\n            if pump3_params(1) > 0\n               P3 = pump3_params(1);\n            elseif not(isempty(pump3_chem))\n               no_errors = 0;\n               error_message = 'Bay 2 Pump 3 flowrate setpoint must be greater than zero';\n            end\n       end\n    end\nelseif Bay2 == 0\n    % .1m bypass\n    Vr2 =length_bypass*D2^2/4*3.14159*1000;\n    if Optimize_params(3)\n          no_errors = 0;\n          error_message = 'Can not optimize temperature on bypass ';\n    end\n\n    if Optimize_params(4)\n       % if user wants to optimize residence time\n        if pump3_params(2) < pump3_params(3)\n             p3_span = [pump3_params(2) ,  pump3_params(3)];\n             p3_span = p3_span;\n             Opt_params(8) = 1;\n         else\n            no_errors = 0;\n            error_message = 'Lower bound of resisdence time must be lower than upper bound';\n        end\n    else\n       if use_flowrate2\n            if P3_setrate < 0\n               no_errors = 0;\n               error_message = 'Pump set flowrates can not be negative';\n            else\n               P3 = P3_setrate;\n            end\n      elseif Bay2_ratio\n           P3 = Bay2_pump_ratio*(P1); % changed from Bay2_pump_ratio*(P1+P2); \n       else\n            if pump3_params(1) > 0\n               P3 = pump3_params(1);\n            elseif not(isempty(pump3_chem))\n               no_errors = 0;\n               error_message = 'Bay 2 Pump 3 setpoint must be greater than zero';\n            end\n       end\n    end\n   else\n    %separator\n    Vr2 = 1000;\n    if Optimize_params(4)\n       % if user wants to optimize residence time\n        if pump3_params(2) < pump3_params(3)\n             p3_span = [pump3_params(2) ,  pump3_params(3)];\n             p3_span = p3_span;\n             Opt_params(8) = 1;\n         else\n            no_errors = 0;\n            error_message = 'Lower bound of pump flowrate must be lower than upper bound';\n        end\n    else\n       if use_flowrate2\n           P3 = P3_setrate;\n       elseif Bay3_ratio\n           P3 = Bay2_pump_ratio*(P1); % changed from Bay2_pump_ratio*(P1+P2); \n       elseif not(isempty(pump3_chem))\n          P3 = 200;\n        end\n      end\n   end\n\n% ****************************************************************************************************\n\n  if Bay3 == 1 \n   %1.05m reactor\n     Vr3= length_reactor1*D3^2/4*3.14159*1000;\n     if  Optimize_params(5)\n       % if choice is made to optimize temperature\n        if T3_params(2) < T3_params(3)\n             T3_span = [T3_params(2) ,  T3_params(3)];\n             Opt_params(3) = 1;\n         else\n            no_errors = 0;\n            error_message = 'Lower bound of temperature must be lower than upper bound';\n        end\n    else\n       %  if choice is made to not optimize temperature\n        T3_SP = T3_params(1);  \n    end\n\n    if Optimize_params(6)\n       % if user wants to optimize residence time\n        if pump4_params(2) < pump4_params(3)\n             p4_span = [pump4_params(2) ,  pump4_params(3)];\n             p4_span = p4_span;\n             Opt_params(9) = 1;\n         else\n            no_errors = 0;\n            error_message = 'Lower bound of pump 4 flowrate must be lower than upper bound';\n        end\n    else\n       if use_flowrate3\n            if P4_setrate < 0\n               no_errors = 0;\n               error_message = 'Pump set flowrates can not be negative';\n            else\n               P4 = P4_setrate;\n            end\n       elseif Bay3_ratio\n            P4= Bay3_pump_ratio*(P1+P2+P3);\n       else\n            if pump4_params(1) > 0\n               %Should a check be made whether or not tau1 > tau2\n                 P4 = pump4_params(1) ;\n            elseif not(isempty(pump4_chem))\n               no_errors = 0;\n               error_message = 'Bay 3 pump 4 setpoint must be greater than zero';\n            end\n       end\n    end\nelseif Bay3 == 0\n    % .1m bypass\n    Vr3 =length_bypass*D3^2/4*3.14159*1000;\n    if Optimize_params(5)\n          no_errors = 0;\n          error_message = 'Can not optimize temperature on bypass ';\n    end\n\n    if Optimize_params(6)\n       % if user wants to optimize residence time\n        if pump4_params(2) < pump4_params(3)\n             p4_span = [pump4_params(2) ,  pump4_params(3)];\n             p4_span = p4_span;\n             Opt_params(9) = 1;\n         else\n            no_errors = 0;\n            error_message = 'Lower bound of pump 4 setpoint must be lower than upper bound';\n        end\n    else\n       if use_flowrate3\n            if P4_setrate < 0\n               no_errors = 0;\n               error_message = 'Pump set flowrates can not be negative';\n            else\n               P4 = P4_setrate;\n            end\n       elseif Bay3_ratio\n            P4= Bay3_pump_ratio*(P1+P2+P3);\n       else\n            if pump4_params(1) > 0\n               P4 =pump4_params(1) ;\n            elseif not(isempty(pump4_chem))\n               no_errors = 0;\n               error_message = 'Bay 3 pump 4 setpoint must be greater than zero';\n            end\n       end\n    end\n   else\n    %separator\n      Vr3 = 1000;\n      if Optimize_params(6)\n       % if user wants to optimize residence time\n        if pump4_params(2) < pump4_params(3)\n             p4_span = [pump4_params(2) ,  pump4_params(3)];\n             p4_span = p4_span;\n             Opt_params(9) = 1;\n         else\n            no_errors = 0;\n            error_message = 'Lower bound of pump 4 flowrate must be lower than upper bound';\n        end\n     else\n        if use_flowrate3\n           P4 = P4_setrate;\n        elseif Bay3_ratio\n            P4= Bay3_pump_ratio*(P1+P2+P3);\n        elseif not(isempty(pump4_chem))\n          P4 = 200;\n        end\n      end\n   end\n\n% ****************************************************************************************************\n\n   if Bay4 == 1 \n   %1.05m reactor\n     Vr4 = length_reactor2*D4^2/4*3.14159*1000;\n     if  Optimize_params(7)\n       % if choice is made to optimize temperature\n        if T4_params(2) < T4_params(3)\n             T4_span = [T4_params(2) ,  T4_params(3)];\n              Opt_params(4) = 1;\n         else\n            no_errors = 0;\n            error_message = 'Lower bound of temperature must be lower than upper bound';\n        end\n    else\n       %  if choice is made to not optimize temperature\n        T4_SP = T4_params(1);  \n    end\n\n    if Optimize_params(8)\n       % if user wants to optimize residence time\n        if pump5_params(2) < pump5_params(3)\n             p5_span = [pump5_params(2) ,  pump5_params(3)];\n             p5_span = p5_span;\n            Opt_params(10) = 1;\n         else\n            no_errors = 0;\n            error_message = 'Lower bound of pump 5 flowrate must be lower than upper bound';\n        end\n    else\n       if use_flowrate4\n            if P5_setrate < 0\n               no_errors = 0;\n               error_message = 'Pump set flowrates can not be negative';\n            else\n               P5 = P5_setrate;\n            end\n       elseif Bay4_ratio\n            P5= Bay4_pump_ratio*(P1+P2+P3+P4);\n       else\n            if pump5_params(1) > 0\n               %Should a check be made whether or not tau4 > tau3\n                 P5 = pump5_params(1) ;\n            elseif not(isempty(pump5_chem))\n               no_errors = 0;\n               error_message = 'Bay 4 Pump 5 setpoint must be greater than zero';\n            end\n       end\n    end\nelseif Bay4 == 0\n    % .1m bypass\n    Vr4 =length_bypass*D4^2/4*3.14159*1000;\n    if Optimize_params(7)\n          no_errors = 0;\n          error_message = 'Can not optimize temperature on bypass ';\n    end\n\n    if Optimize_params(8)\n       % if user wants to optimize residence time\n        if pump5_params(2) < pump5_params(3)\n             p5_span = [pump5_params(2) ,  pump5_params(3)];\n             p5_span = p5_span;\n             Opt_params(10) = 1;\n         else\n            no_errors = 0;\n            error_message = 'Lower bound of resisdence time must be lower than upper bound';\n        end\n    else\n       if use_flowrate4\n            if P5_setrate < 0\n               no_errors = 0;\n               error_message = 'Pump set flowrates can not be negative';\n            else\n               P5 = P5_setrate;\n            end\n       elseif Bay4_ratio\n            P5= Bay4_pump_ratio*(P1+P2+P3+P4);\n       else\n            if pump5_params(1) > 0\n               P5 = pump5_params(1);\n            elseif not(isempty(pump5_chem))\n               no_errors = 0;\n               error_message = 'Bay 4 pump 5 setpoint must be greater than zero';\n            end\n       end\n    end\n   else\n    %separator\n      Vr4 = 1000;\n      if Optimize_params(8)\n       % if user wants to optimize residence time\n         if pump5_params(2) < pump5_params(3)\n             p5_span = [pump5_params(2) ,  pump5_params(3)];\n             p5_span = p5_span;\n             Opt_params(10) = 1;\n         else\n            no_errors = 0;\n            error_message = 'Lower bound of resisdence time must be lower than upper bound';\n         end\n       else\n           if use_flowrate4\n              P5 = P5_setrate;\n           elseif Bay4_ratio\n              P5= Bay4_pump_ratio*(P1+P2+P3+P4);\n           elseif not(isempty(pump5_chem))\n              P5 = 200;\n           end\n        end\n   end\n\n% ****************************************************************************************************\n\n  if Bay5 == 1 \n   %1.05m reactor\n     Vr5= length_reactor*D5^2/4*3.14159*1000;\n     if  Optimize_params(9)\n       % if choice is made to optimize temperature\n        if T5_params(2) < T5_params(3)\n             T5_span = [T5_params(2) ,  T5_params(3)];\n             Opt_params(5) = 1;\n         else\n            no_errors = 0;\n            error_message = 'Lower bound of temperature must be lower than upper bound';\n        end\n    else\n       %  if choice is made to not optimize temperature\n        T5_SP = T5_params(1);  \n    end\n\n    if Optimize_params(10)\n       % if user wants to optimize residence time\n        if pump6_params(2) < pump6_params(3)\n             p6_span = [pump6_params(2) ,  pump6_params(3)];\n             p6_span = p6_span;\n             Opt_params(11) = 1;\n         else\n            no_errors = 0;\n            error_message = 'Lower bound of pump 6 flowrate must be lower than upper bound';\n        end\n    else\n       if use_flowrate5\n            if P6_setrate < 0\n               no_errors = 0;\n               error_message = 'Pump set flowrates can not be negative';\n            else\n               P6 = P6_setrate;\n            end\n      elseif Bay5_ratio\n              P6= Bay5_pump_ratio*(P1+P2+P3+P4+P5);\n      else\n            if pump6_params(1) > 0\n               %Should a check be made whether or not tau1 > tau2\n                 P6 =pump6_params(1) ;\n            elseif not(isempty(pump6_chem))\n               no_errors = 0;\n               error_message = 'Bay 5 pump 6 setpoint must be greater than zero';\n            end\n       end\n    end\nelseif Bay5 == 0\n    % .1m bypass\n    Vr5 =length_bypass*D5^2/4*3.14159*1000;\n    if Optimize_params(9)\n          no_errors = 0;\n          error_message = 'Can not optimize temperature on bypass ';\n    end\n\n    if Optimize_params(10)\n       % if user wants to optimize residence time\n        if pump6_params(2) < pump6_params(3)\n             p6_span = [pump6_params(2) ,  pump6_params(3)];\n             p6_span = p6_span;\n             Opt_params(11) = 1;\n         else\n            no_errors = 0;\n            error_message = 'Lower bound of pump 6 must be lower than upper bound';\n        end\n    else\n       if use_flowrate5\n            if P6_setrate < 0\n               no_errors = 0;\n               error_message = 'Pump set flowrates can not be negative';\n            else\n               P6 = P6_setrate;\n            end\n      elseif Bay5_ratio\n              P6= Bay5_pump_ratio*(P1+P2+P3+P4+P5);\n       else\n            if pump6_params(1) > 0\n               P6 = pump6_params(1);\n            elseif not(isempty(pump6_chem))\n               no_errors = 0;\n               error_message = 'Bay 5 pump 6 setpoint must be greater than zero';\n            end\n       end\n    end\n   else\n    %separator\n      Vr5 = 1000;\n      if Optimize_params(10)\n       % if user wants to optimize residence time\n        if pump6_params(2) < pump6_params(3)\n             p6_span = [pump6_params(2) ,  pump6_params(3)];\n             p6_span = p6_span;\n             Opt_params(11) = 1;\n         else\n            no_errors = 0;\n            error_message = 'Lower bound of pump 6 must be lower than upper bound';\n        end\n      else\n         if use_flowrate5\n               P6 = P6_setrate;\n         elseif Bay5_ratio\n               P6= Bay5_pump_ratio*(P1+P2+P3+P4+P5);\n         elseif not(isempty(pump6_chem))\n              P6 = 200;\n         end\n      end\n   end\n\n% ****************************************************************************************************\n\n%Setup optimization\n\n   initialize_opt = 0;\n\n%*****************************************************************************************************\n% Setup excel and xml file writing\n\npath(path, pa);\nnumMSSig = 1;\n\n%Setup output excel file\n% Opening Excel file and inputing first peaks headers if needed\ntry\n  xlApp = actxGetRunningServer('Excel.Application');\ncatch ME\n  xlApp = actxserver('Excel.Application');\nend\n\nxlApp.DisplayAlerts = false; \nxlApp.Visible = false;\n\n%try\n   xlWorkbook = xlApp.workbooks.Open(xl_file, 0,false);\n   xlSheets = xlWorkbook.Sheets;\n   xlSheetNamesArray = cell(xlSheets.Count, 1);\n\n  for i = 1:xlSheets.Count\n     xlSheetNamesArray{i} = xlSheets.Item(i).Name;\n  end\n\n  [~, idx1] = ismember('Time_Series_Conditions', xlSheetNamesArray);\n  lastcol1 = xlcolumnletter(22);\n\n  [~, idx2] = ismember('MS Results', xlSheetNamesArray);\n  lastcol2 = xlcolumnletter(2);\n\n  [~, idx3] = ismember('System Setup', xlSheetNamesArray);\n  lastcol3 = xlcolumnletter(11);\n\n  [~, idx4] = ismember('HPLC Results', xlSheetNamesArray);\n  lastcol4 = xlcolumnletter(3);\n\n  [~, idx_ir_exp] = ismember('IR Results', xlSheetNamesArray);\n  IR_i= xlSheets.Item(idx_ir_exp).Range('A1').End('xlDown').Row ; \n  if IR_i == 1048576\n     IR_i = 2;\n  end\n \n  lastrow1 =  xlSheets.Item(idx1).Range('A1').End('xlDown').Row;\n  if lastrow1 == 1048576\n      lastrow1 = 2;\n  end\n\n  lastrow2 =  xlSheets.Item(idx2).Range('A1').End('xlDown').Row;\n  if lastrow2 == 1048576\n      lastrow2 = 2;\n  end\n\n   lastrow3= 2;\n\n    lastrow4=  xlSheets.Item(idx4).Range('A1').End('xlDown').Row;\n    if lastrow4 == 1048576\n       lastrow4 =2;\n    end\n\n%catch ME\n %   xlWorkbook = xlApp.Workbooks;\n %  xlWorkbook = invoke(xlWorkbook, 'Add');\n %   WS = xlWorkbook.Worksheets;\n %   row = num2str(1);\n %   temp_write = [Bay1, Bay2, Bay3, Bay4, Bay5, 1, Vr1, Vr2, Vr3, Vr4, Vr5];\n %   xlSheets.Item(idx3).Range(strcat('A',row,':',lastcol3,row)).Value2 =  temp_write;\n %   WS.Add([], WS.Item(WS.Count));\n %   WS.Item(WS.Count).Name = 'Time_Series_Conditions';\n %    WS.Add([], WS.Item(WS.Count));\n %    WS.Item(WS.Count).Name = 'MS Results';\n %   WS.Add([], WS.Item(WS.Count));\n %    WS.Item(WS.Count).Name = 'System Setup';\n %   WS.Add([], WS.Item(WS.Count));\n %    WS.Item(WS.Count).Name = 'HPLC Results';\n%end\n\nload('C:\\Users\\HPLC\\Dropbox (MIT)\\MoD Files\\MATLAB\\IR_Pks.mat');\n\ntemp_write = [Bay1, Bay2, Bay3, Bay4, Bay5, 1, Vr1, Vr2, Vr3, Vr4, Vr5];\nlastrowStr3 = num2str(lastrow3);\nxlSheets.Item(idx3).Range(strcat('A',lastrowStr3,':',lastcol3,lastrowStr3)).Value2 =  temp_write;\nlastrow3 = lastrow3 +1;\n\ntemp_write = {pump1_chem, pump2_chem, pump3_chem, pump4_chem, pump5_chem, pump6_chem};\nlastrowStr3 = num2str(6);\nxlSheets.Item(idx3).Range(strcat('B',lastrowStr3,':','G',lastrowStr3)).Value2 =  temp_write;\n\nlastrowStr3 = num2str(8);\nxlSheets.Item(idx3).Range(strcat('B',lastrowStr3,':','G',lastrowStr3)).Value2 = Pump_concen;\n\n\n\n%***************************************************************************************************\n\nredo = false;\nncall = ncall_in;"("Bay1"=w362, "Bay2"=w361, "Bay3"=w360, "Bay4"=w359, "Bay5"=w358, "tube_id"=w357, "use_flowrate1"=w344, "P1_setrate"=w356, "P2_setrate"=w355, "P3_setrate"=w354, "P4_setrate"=w353, "P5_setrate"=w352, "P6_setrate"=w351, "use_flowrate2"=w294, "use_flowrate3"=w341, "use_flowrate4"=w340, "use_flowrate5"=w337, "Optimize_params"=w316, "T1_params"=w313, "T2_params"=w312, "T3_params"=w311, "T4_params"=w310, "T5_params"=w309, "pump1_params"=w308, "pump3_params"=w307, "pump4_params"=w306, "pump5_params"=w305, "pump6_params"=w304, "P1_P2_ratio"=w301, "xml_file"=w300, "xl_file"=w299, "pa"=w298, "Continue"=w296, "matlabsavefile"=w295, "Bay2_ratio"=w292, "Bay2_pump_ratio"=w291, "Bay3_ratio"=w289, "Bay3_pump_ratio"=w288, "Bay4_ratio"=w286, "Bay4_pump_ratio"=w285, "Bay5_ratio"=w283, "Bay5_pump_ratio"=w282, "pump1_chem"=w274, "pump6_chem"=w273, "pump5_chem"=w272, "pump4_chem"=w271, "pump3_chem"=w270, "pump2_chem"=w269, "Pump_concen"=w262, "pump2_params"=w260) -> ("Vr1"=w350:dbl, "Vr2"=w349:dbl, "Vr3"=w348:dbl, "Vr4"=w347:dbl, "Vr5"=w346:dbl, "no_errors"=w315:dbl, "error_message"=w314:string)  [unwired: 1 in, 1 out]
                        n218 = Not Equal To 0?(x=w315) -> (x != 0?=w302:bool)
                        n219 = Not(x=w302) -> (.not. x?=w303:bool)
                        n220 = case shown="True" w303 {
                          tunnel: w314 -> [_ w363]
                          frame False {
                          }
                          frame True {
                            n221 = One Button Dialog(message=w363) -> ()  [unwired: 1 in, 1 out]
                          }
                        }
                      }
                    }
                    n222 = local read "Stop"() -> (w235:bool)
                    n223 = Or(x=w227, y=w235) -> (x .or. y?=w236:bool)
                    n224 = Wait (ms)(milliseconds to wait=u32 500) -> ()  [unwired: 1 out]
                  }
                  n225 = local write "Volume (ul) 1"(w221) -> ()
                  n226 = local write "Volume (ul) 2"(w220) -> ()
                  n227 = local write "Volume (ul) 3"(w219) -> ()
                  n228 = local write "Volume (ul) 4"(w218) -> ()
                  n229 = local write "Volume (ul) 5"(w217) -> ()
                }
                frame #2 {
                  n230 = local write "Paramter Confirm"(w364) -> ()
                }
              }
            }
          }
        }
        frame #2 {
          # "Run Initial diagnostics"
        }
        frame #3 {
          # "Run System"
          n231 = while {
            stop <- w824 stop-if-true
            n232 = local read "Debug_run_button"() -> (w820:bool)
            n233 = Not(x=w820) -> (.not. x?=w822:bool)
            n234 = local read "Temperature Control 1"() -> (w819:bool)
            n235 = And(x=w822, y=w819) -> (x .and. y?=w821:bool)
            n236 = case shown="True" w821 {
              frame False {
                n237 = local write "Temp SS? 1"(TRUE ("Temp SS? 1")) -> ()
              }
              frame True {
                # "Bay 1 Temperature Controller"
                n238 = local read "Temperature SP 1"() -> (w826:dbl)
                n239 = local read "Temperature 1"() -> (w827:dbl)
                n240 = local read "SSR Duration 1"() -> (w837:dbl)
                n241 = call-poly <vilib>:"PID Online Autotuning.vi"("setpoint"=w826, "manipulated variable"=w837, "autotuning parameters"=T8 {"type of controller"=enum."PID", "relay cycles"=3, "relay amplitude"=1.0, "control specifications"=enum."Normal", "PV noise level"=0.1} ("Autotuning Parameters R1"), "process variable"=w827, "PID gains in"=T7 {"Proportional gain Kc"=0.38538, "Integral time Ti (sec)"=0.524375, "Derivative time Ti (sec)"=0.12585} ("PID gains 2")) -> ("setpoint out"=w843:dbl, "process variable out"=w842:dbl, "PID gains out"=w839:T9)  [unwired: 6 in, 2 out]
                n242 = call <vilib>:"PID Autotuning (Temperature).vi"("desired temperature"=w843, "measured temperature"=w842, "plant parameters in"=w839, "output range"=cluster{"output high":dbl, "output low":dbl} {"output high"=3.0, "output low"=-1.0} ("Output range")) -> ("output"=w835:dbl)  [unwired: 12 in, 3 out]
                n243 = local write "SSR Duration 1"(w835) -> ()
                n244 = Subtract(x=w826, y=w827) -> (x-y=w828:dbl)
                n245 = Absolute Value(x=w828) -> (abs(x)=w831:dbl)
                n246 = Multiply(x=1000.0, y=w835) -> (x*y=w833:dbl)
                n247 = Greater Than 0?(x=w833) -> (x > 0?=w832:bool)
                n248 = Less Or Equal?(x=w831, y=1.2) -> (x <= y?=w829:bool)
                n249 = case shown="False" w832 {
                  tunnel: 2 -> [_ _]
                  tunnel: w833 -> [w844 _]
                  frame False {
                    (unwired) errorcluster {"status"=FALSE, "code"=0, "source"=""} ("error out")
                    n250 = Absolute Value(x=w844) -> (abs(x)=w845:dbl)
                    n251 = Wait (ms)(milliseconds to wait=w845) -> ()  [unwired: 1 out]
                  }
                  frame True {
                  }
                }
                n252 = local write "Temp SS? 1"(w829) -> ()
              }
            }
            n253 = Wait (ms)(milliseconds to wait=u32 300) -> ()  [unwired: 1 out]
            n254 = local read "Stop"() -> (w824:bool)
          }
          n255 = local read "Bay Parameters"() -> (w367:T4)
          n256 = while {
            stop <- w797 stop-if-true
            n257 = local read "Debug_run_button"() -> (w793:bool)
            n258 = Not(x=w793) -> (.not. x?=w795:bool)
            n259 = local read "Temperature Control 2"() -> (w792:bool)
            n260 = And(x=w795, y=w792) -> (x .and. y?=w794:bool)
            n261 = case shown="True" w794 {
              frame False {
                n262 = local write "Temp SS? 2"(TRUE ("Temp SS? 2")) -> ()
              }
              frame True {
                # "Bay 2 Temperature Controller"
                n263 = local read "Temperature SP 2"() -> (w800:dbl)
                n264 = local read "Temperature 2"() -> (w799:dbl)
                n265 = local read "SSR Duration 2"() -> (w813:dbl)
                n266 = call-poly <vilib>:"PID Online Autotuning.vi"("setpoint"=w800, "manipulated variable"=w813, "autotuning parameters"=T8 {"type of controller"=enum."PID", "relay cycles"=3, "relay amplitude"=1.0, "control specifications"=enum."Normal", "PV noise level"=0.1} ("Autotuning Parameters R1"), "process variable"=w799, "PID gains in"=T7 {"Proportional gain Kc"=0.38538, "Integral time Ti (sec)"=0.524375, "Derivative time Ti (sec)"=0.12585} ("PID gains 2")) -> ("setpoint out"=w811:dbl, "process variable out"=w810:dbl, "PID gains out"=w816:T9)  [unwired: 6 in, 2 out]
                n267 = call <vilib>:"PID Autotuning (Temperature).vi"("desired temperature"=w811, "measured temperature"=w810, "plant parameters in"=w816, "output range"=cluster{"output high":dbl, "output low":dbl} {"output high"=3.0, "output low"=-1.0} ("Output range")) -> ("output"=w805:dbl)  [unwired: 12 in, 3 out]
                n268 = local write "SSR Duration 2"(w805) -> ()
                n269 = Multiply(x=1000.0, y=w805) -> (x*y=w807:dbl)
                n270 = Greater Than 0?(x=w807) -> (x > 0?=w808:bool)
                n271 = case shown="False" w808 {
                  tunnel: 3 -> [_ _]
                  tunnel: w807 -> [w817 _]
                  frame False {
                    (unwired) errorcluster {"status"=FALSE, "code"=0, "source"=""} ("error out")
                    n272 = Absolute Value(x=w817) -> (abs(x)=w818:dbl)
                    n273 = Wait (ms)(milliseconds to wait=w818) -> ()  [unwired: 1 out]
                  }
                  frame True {
                  }
                }
                n274 = Subtract(x=w800, y=w799) -> (x-y=w802:dbl)
                n275 = Absolute Value(x=w802) -> (abs(x)=w804:dbl)
                n276 = Less Or Equal?(x=w804, y=1.2) -> (x <= y?=w801:bool)
                n277 = local write "Temp SS? 2"(w801) -> ()
              }
            }
            n278 = local read "Stop"() -> (w797:bool)
            n279 = Wait (ms)(milliseconds to wait=u32 300) -> ()  [unwired: 1 out]
          }
          n280 = local read "Stop"() -> (w365:bool)
          n281 = Not(x=w365) -> (.not. x?=w366:bool)
          n282 = case shown="True" w366 {
            tunnel: w367 -> [_ w368]
            frame False {
            }
            frame True {
              n283 = while {
                tunnel: w368 -> [w379]
                i -> [w378]
                stop <- w370 stop-if-true
                n284 = local read "Debug_run_button"() -> (w381:bool)
                n285 = Wait (ms)(milliseconds to wait=u32 1000) -> ()  [unwired: 1 out]
                n286 = Increment(x=w378) -> (x+1=w377:i32)
                n287 = case shown="False" w381 {
                  tunnel: w378 -> [_ w693]
                  tunnel: w379 -> [_ _]
                  tunnel: [200.0 w695] -> w374
                  tunnel: [w391 0.0] -> w372
                  frame False {
                    # "SNOBFIT"
                    # "Optimize"
                    # "Run Experimental Conditions"
                    # "Optimize/Synthesize"
                    n288 = script code="if not(redo)\n    % snobfit\n    snobfit_labview_driver;\nend"() -> ("??"=w384:errorcluster)  [unwired: 1 in]
                    n289 = flat-sequence {
                      tunnel: w384 -> [w399]
                      tunnel: [w399] -> w383
                      frame #0 {
                        n290 = One Button Dialog(message="Click Ok 1") -> ()  [unwired: 1 in, 1 out]
                      }
                    }
                    n291 = script code="if not(system_error)\nif not(redo)\n    % snobfit\n    %snobfit_labview_driver;\n\n    if opt_ctr == 2\n      new_x = x(req_ctr,:);\n      x_ind = 1;\n      \n      if Opt_params(1)\n         T1_SP = new_x(x_ind ); %'C\n         params_1(1) = new_x(x_ind);\n         x_ind  = x_ind  + 1;\n      end\n     if Opt_params(2)\n       T2_SP = new_x(x_ind ); %'C\n        params_1(3) = new_x(x_ind);\n       x_ind  = x_ind  + 1;\n     end\n     if Opt_params(3)\n       T3_SP = new_x(x_ind ); %'C\n       x_ind  = x_ind  + 1;\n    end\n     if Opt_params(4)\n       T4_SP = new_x(x_ind ); %'C\n       x_ind  = x_ind  + 1;\n    end\n     if Opt_params(5)\n       T5_SP = new_x(x_ind ); %'C\n       x_ind  = x_ind  + 1;\n    end\n    if Opt_params(6)\n        tau1 = Vr1/(new_x( x_ind) +new_x( x_ind+1) );\n        %new_x( x_ind) = tau1*60;\n        params_1(2) = new_x(x_ind);\n        P2 =new_x( x_ind+1); %ul/min\n        P1=new_x( x_ind); %ul/min\n        x_ind  = x_ind  + 2;\n    end\n     if Opt_params(8)\n        tau2= Vr2/(new_x( x_ind)+P1+P2);\n        %new_x( x_ind) = tau2*60;\n        params_1(4) = new_x(x_ind);\n        P3=new_x( x_ind); %ul/minP2 = Vr4/(tau4)*60/2;\n        x_ind  = x_ind  + 1;\n      % P2 = Vr4/(tau4)*60/2;\n     elseif Bay2_ratio && not(use_flowrate2)\n        P3= Bay2_pump_ratio*(P1+P2); %chnaged from  P3= Bay2_pump_ratio*(P1 + P2);\n      end\n    if Opt_params(9)\n      tau3 =Vr3/(new_x( x_ind)+P1+P2+P3);\n      P4=new_x( x_ind); %ul/min\n      P3= Bay2_pump_ratio*(P4); \n      x_ind  = x_ind  + 1;\n    elseif Bay3_ratio && not(use_flowrate3)\n        P4= Bay3_pump_ratio*(P1+P2 +P3);\n    end\n    if Opt_params(10)\n      tau4 = Vr4/(new_x( x_ind)+P1+P2+P3+P4);\n      P5=new_x( x_ind) ; %ul/min\n       x_ind  = x_ind  + 1;\n    elseif Bay4_ratio && not(use_flowrate4)\n        P5= Bay4_pump_ratio*(P1+P2 +P3 +P4);\n    end\n    if Opt_params(11)\n      tau5 = Vr5/(new_x( x_ind)+P1+P2+P3+P4+P5);\n      %new_x( x_ind) = tau5*60;\n      P6=new_x( x_ind) ; %ul/min\n      x_ind  = x_ind  + 1;\n    elseif Bay5_ratio && not(use_flowrate5)\n        P6= Bay5_pump_ratio*(P1+P2 +P3 +P4 +P4 +P5);\n    end\n    %---------  \n end\n\n   %P2 =P2 /2;\n   Conditions_Array = [P1 P2/2 P3 P4 P5 P6 T1_SP T2_SP T3_SP T4_SP T5_SP];\n   if opt_ctr == 2\n        opt_ctr = 1;\n   else\n       opt_ctr = 2\n   end\nelse\n   opt_ctr =1;\n   redo = false;\n   if req_ctr ~= req_tot\n       req_ctr = req_ctr - 1;\n   end\n   CurrExp = CurrExp - 1;\n   ncall0 = ncall0 - 1;\n end\n\nend\n\nP_tot = P1 + P2 + P3 + P4 + P5 + P6 ;"("??"=w383) -> ("Conditions_Array"=w386:dbl[], "opt_ctr"=w396:dbl)  [unwired: 1 out]
                    n292 = local read "COMM Port :: Milligat Pumps"() -> (w397:refnum<visa-resource-name>)
                    n293 = Equal?(x=w396, y=1.0) -> (x = y?=w394:bool)
                    n294 = flat-sequence {
                      tunnel: w386 -> [w641]
                      frame #0 {
                        n295 = Index Array(array=w641, index=5) -> (element=w658:dbl)
                        n296 = Index Array(array=w641, index=0) -> (element=w650:dbl)
                        n297 = Index Array(array=w641, index=1) -> (element=w651:dbl)
                        n298 = Index Array(array=w641, index=2) -> (element=w656:dbl)
                        n299 = Index Array(array=w641, index=3) -> (element=w655:dbl)
                        n300 = Index Array(array=w641, index=4) -> (element=w657:dbl)
                        n301 = local read "Volume (ul) 3"() -> (w628:dbl)
                        n302 = local read "Volume (ul) 5"() -> (w626:dbl)
                        n303 = local read "Volume (ul) 4"() -> (w627:dbl)
                        n304 = local read "Volume (ul) 2"() -> (w629:dbl)
                        n305 = local read "Volume (ul) 1"() -> (w630:dbl)
                        n306 = local write "stop_xl_write"(FALSE ("stop_xl_write")) -> ()
                        n307 = Add(x=w650, y=w651) -> (x+y=w639:dbl)
                        n308 = Add(x=w639, y=w656) -> (x+y=w637:dbl)
                        n309 = Add(x=w637, y=w655) -> (x+y=w635:dbl)
                        n310 = Add(x=w635, y=w657) -> (x+y=w632:dbl)
                        n311 = Add(x=w632, y=w658) -> (x+y=w634:dbl)
                        n312 = local write "Pump setpoint(ul/min) 2"(w651) -> ()
                        n313 = local write "Pump setpoint(ul/min) 4"(w656) -> ()
                        n314 = local write "Pump setpoint(ul/min) 5"(w657) -> ()
                        n315 = Not Equal To 0?(x=w639) -> (x != 0?=w640:bool)
                        n316 = local write "Pump setpoint(ul/min) 3"(w655) -> ()
                        n317 = local write "Pump setpoint(ul/min) 6"(w658) -> ()
                        n318 = local write "Pump setpoint(ul/min) 1"(w650) -> ()
                        n319 = Not Equal To 0?(x=w634) -> (x != 0?=w631:bool)
                        n320 = Not Equal To 0?(x=w635) -> (x != 0?=w636:bool)
                        n321 = Not Equal To 0?(x=w632) -> (x != 0?=w633:bool)
                        n322 = Not Equal To 0?(x=w637) -> (x != 0?=w638:bool)
                        n323 = case shown="True" w638 {
                          tunnel: w637 -> [_ w674]
                          tunnel: [0.0 w673] -> w649
                          tunnel: w629 -> [_ w672]
                          frame False {
                          }
                          frame True {
                            n324 = Divide(x=w672, y=w674) -> (x/y=w673:dbl)
                          }
                        }
                        n325 = case shown="True" w631 {
                          tunnel: w634 -> [_ w666]
                          tunnel: [0.0 w665] -> w654
                          tunnel: w626 -> [_ w664]
                          frame False {
                          }
                          frame True {
                            n326 = Divide(x=w664, y=w666) -> (x/y=w665:dbl)
                          }
                        }
                        n327 = case shown="True" w636 {
                          tunnel: [0.0 w670] -> w652
                          tunnel: w635 -> [_ w669]
                          tunnel: w628 -> [_ w668]
                          frame False {
                          }
                          frame True {
                            n328 = Divide(x=w668, y=w669) -> (x/y=w670:dbl)
                          }
                        }
                        n329 = case shown="True" w640 {
                          tunnel: w639 -> [_ w678]
                          tunnel: [0.0 w677] -> w648
                          tunnel: w630 -> [_ w676]
                          frame False {
                          }
                          frame True {
                            n330 = Divide(x=w676, y=w678) -> (x/y=w677:dbl)
                          }
                        }
                        n331 = case shown="True" w633 {
                          tunnel: w632 -> [_ w662]
                          tunnel: [0.0 w661] -> w653
                          tunnel: w627 -> [_ w660]
                          frame False {
                          }
                          frame True {
                            n332 = Divide(x=w660, y=w662) -> (x/y=w661:dbl)
                          }
                        }
                        n333 = local write "tau 2"(w649) -> ()
                        n334 = local write "tau 3"(w652) -> ()
                        n335 = local write "tau 4"(w653) -> ()
                        n336 = local write "tau 5"(w654) -> ()
                        n337 = local write "tau 1"(w648) -> ()
                      }
                    }
                    n338 = flat-sequence {
                      tunnel: w397 -> [w406]
                      tunnel: w386 -> [w405]
                      tunnel: w394 -> [w404]
                      tunnel: [w404] -> w393
                      tunnel: w393 -> [w495]
                      tunnel: [w495] -> w392
                      tunnel: w392 -> [w511]
                      tunnel: w386 -> [w541]
                      tunnel: [w540] -> w385
                      tunnel: [w581] -> w389
                      tunnel: w385 -> [_]
                      tunnel: w389 -> [w585]
                      tunnel: [w585] -> w388
                      tunnel: w388 -> [w593]
                      tunnel: [w593] -> w387
                      tunnel: [w624] -> w391
                      tunnel: w387 -> [w624]
                      frame #0 {
                        # "Setup pump flowrates and temperature setpoints"
                        n339 = stacked-sequence {
                          tunnel: w406 -> [w422 _ _ _ _]
                          tunnel: w406 -> [_ w440 _ _ _]
                          tunnel: w406 -> [_ _ w456 _ _]
                          tunnel: w406 -> [_ _ _ w472 _]
                          tunnel: w406 -> [_ _ _ _ w490]
                          tunnel: w405 -> [w419 w438 w454 w470 w485]
                          tunnel: w404 -> [w408 w430 w446 w462 w478]
                          frame #0 {
                            # "Bay 1"
                            n340 = local read "Syringe_pump?"() -> (w407:bool)
                            n341 = Index Array(array=w419, index=0) -> (element=w417:dbl)
                            n342 = local read "Bay 1"() -> (w424:u16)
                            n343 = Index Array(array=w419, index=1) -> (element=w416:dbl)
                            n344 = Index Array(array=w419, index=6) -> (element=w415:dbl)
                            n345 = script code="MATLAB script"("P1"=w417, "P2"=w416, "T1_SP"=w415) -> ()  [unwired: 1 in, 1 out]
                            n346 = Greater Than 0?(x=w417) -> (x > 0?=w414:bool)
                            n347 = And(x=w414, y=w408) -> (x .and. y?=w413:bool)
                            n348 = Equal?(x=w424, y=u16 1) -> (x = y?=w410:bool)
                            n349 = Greater Than 0?(x=w416) -> (x > 0?=w412:bool)
                            n350 = And(x=w412, y=w408) -> (x .and. y?=w411:bool)
                            n351 = And(x=w410, y=w408) -> (x .and. y?=w409:bool)
                            n352 = case shown="True" w407 {
                              tunnel: w422 -> [_ _]
                              tunnel: w416 -> [w426 _]
                              tunnel: w411 -> [w425 w427]
                              frame False {
                                n353 = case shown="True" w425 {
                                tunnel: w426 -> [_ _]
                                frame False {
                                }
                                frame True {
                                }
                                }
                              }
                              frame True {
                                n354 = case shown="False" w427 {
                                frame False {
                                }
                                frame True {
                                }
                                }
                              }
                            }
                            n355 = case shown="True" w413 {
                              tunnel: w422 -> [_ _]
                              tunnel: w417 -> [_ _]
                              frame False {
                              }
                              frame True {
                                # "switched j and g"
                              }
                            }
                            n356 = case shown="True" w409 {
                              tunnel: w415 -> [_ w429]
                              frame False {
                                n357 = local write "Temperature Control 1"(FALSE) -> ()
                              }
                              frame True {
                                n358 = local write "Temperature SP 1"(w429) -> ()
                              }
                            }
                          }
                          frame #1 {
                            # "Bay 2"
                            n359 = Index Array(array=w438, index=2) -> (element=w435:dbl)
                            n360 = Index Array(array=w438, index=7) -> (element=w436:dbl)
                            n361 = script code="MATLAB script"("T2_SP"=w436, "P3"=w435) -> ()  [unwired: 1 in, 1 out]
                            n362 = local read "Bay 2"() -> (w441:u16)
                            n363 = Equal?(x=w441, y=u16 1) -> (x = y?=w434:bool)
                            n364 = Greater Than 0?(x=w435) -> (x > 0?=w432:bool)
                            n365 = And(x=w434, y=w430) -> (x .and. y?=w433:bool)
                            n366 = And(x=w432, y=w430) -> (x .and. y?=w431:bool)
                            n367 = case shown="True" w433 {
                              tunnel: w436 -> [_ w444]
                              frame False {
                                n368 = local write "Temperature Control 2"(FALSE) -> ()
                              }
                              frame True {
                                n369 = local write "Temperature Control 2"(TRUE ("Temperature Control 2")) -> ()
                                n370 = local write "Temperature SP 2"(w444) -> ()
                              }
                            }
                            n371 = case shown="False" w431 {
                              tunnel: w435 -> [_ _]
                              tunnel: w440 -> [_ _]
                              frame False {
                              }
                              frame True {
                              }
                            }
                          }
                          frame #2 {
                            # "Bay 3"
                            n372 = Index Array(array=w454, index=3) -> (element=w451:dbl)
                            n373 = local read "Bay 3"() -> (w458:u16)
                            n374 = Not Equal To 0?(x=w451) -> (x != 0?=w450:bool)
                            n375 = Index Array(array=w454, index=8) -> (element=w452:dbl)
                            n376 = script code="MATLAB script"("T3_SP"=w452, "P4"=w451) -> ()  [unwired: 1 in, 1 out]
                            n377 = Equal?(x=w458, y=u16 1) -> (x = y?=w448:bool)
                            n378 = And(x=w448, y=w446) -> (x .and. y?=w447:bool)
                            n379 = And(x=w450, y=w446) -> (x .and. y?=w449:bool)
                            n380 = case shown="True" w447 {
                              tunnel: w452 -> [_ w460]
                              frame False {
                                n381 = local write "Temperature Control 3"(FALSE) -> ()
                              }
                              frame True {
                                n382 = local write "Temperature Control 3"(TRUE ("Temperature Control 3")) -> ()
                                n383 = local write "Temperature SP 3"(w460) -> ()
                              }
                            }
                            n384 = case shown="True" w449 {
                              tunnel: w451 -> [_ _]
                              tunnel: w456 -> [_ _]
                              frame False {
                              }
                              frame True {
                              }
                            }
                          }
                          frame #3 {
                            # "Bay 4"
                            n385 = Index Array(array=w470, index=9) -> (element=w467:dbl)
                            n386 = Index Array(array=w470, index=4) -> (element=w468:dbl)
                            n387 = script code="MATLAB script"("P5"=w468, "T4_SP"=w467) -> ()  [unwired: 1 in, 1 out]
                            n388 = Not Equal To 0?(x=w468) -> (x != 0?=w466:bool)
                            n389 = local read "Bay 4"() -> (w473:u16)
                            n390 = Equal?(x=w473, y=1) -> (x = y?=w463:bool)
                            n391 = And(x=w466, y=w462) -> (x .and. y?=w465:bool)
                            n392 = And(x=w463, y=w462) -> (x .and. y?=w464:bool)
                            n393 = case shown="False" w465 {
                              tunnel: w472 -> [_ _]
                              tunnel: w468 -> [_ _]
                              frame False {
                              }
                              frame True {
                              }
                            }
                            n394 = case shown="True" w464 {
                              tunnel: w467 -> [_ w476]
                              frame False {
                                n395 = local write "Temperature Control 4"(FALSE ("Temperature Control 4")) -> ()
                              }
                              frame True {
                                n396 = local write "Temperature SP 4"(w476) -> ()
                                n397 = local write "Temperature Control 4"(TRUE ("Temperature Control 5")) -> ()
                              }
                            }
                          }
                          frame #4 {
                            # "Bay 5"
                            n398 = Index Array(array=w485, index=5) -> (element=w483:dbl)
                            n399 = Index Array(array=w485, index=4) -> (element=w484:dbl)
                            n400 = script code="MATLAB script"("T5_SP"=w484, "P6"=w483) -> ()  [unwired: 1 in, 1 out]
                            n401 = Not Equal To 0?(x=w483) -> (x != 0?=w480:bool)
                            n402 = And(x=w480, y=w478) -> (x .and. y?=w479:bool)
                            n403 = local read "Bay 5"() -> (w489:u16)
                            n404 = Equal?(x=w489, y=u16 1) -> (x = y?=w481:bool)
                            n405 = And(x=w481, y=w478) -> (x .and. y?=w482:bool)
                            n406 = case shown="True" w482 {
                              tunnel: w484 -> [_ w492]
                              frame False {
                                n407 = local write "Temperature Control 5"(FALSE ("Temperature Control 5")) -> ()
                              }
                              frame True {
                                n408 = local write "Temperature SP 5"(w492) -> ()
                                n409 = local write "Temperature Control 5"(TRUE ("Temperature Control 5")) -> ()
                              }
                            }
                            n410 = case shown="True" w479 {
                              tunnel: w490 -> [_ _]
                              tunnel: w483 -> [_ _]
                              frame False {
                              }
                              frame True {
                              }
                            }
                          }
                        }
                      }
                      frame #1 {
                        # "Wait till Steady State temperature readings on all bays"
                        n411 = while {
                          tunnel: w495 -> [w498]
                          stop <- w508 stop-if-true
                          n412 = local read "Temp SS? 2"() -> (w505:bool)
                          n413 = local read "Temp SS? 3"() -> (w504:bool)
                          n414 = local read "Temp SS? 4"() -> (w503:bool)
                          n415 = local read "Temp SS? 5"() -> (w502:bool)
                          n416 = local read "Temp SS? 1"() -> (w506:bool)
                          n417 = Wait (ms)(milliseconds to wait=u32 1500) -> ()  [unwired: 1 out]
                          n418 = local read "Stop"() -> (w507:bool)
                          n419 = And(x=w504, y=w503) -> (x .and. y?=w500:bool)
                          n420 = And(x=w506, y=w505) -> (x .and. y?=w499:bool)
                          n421 = And(x=w499, y=w500) -> (x .and. y?=w501:bool)
                          n422 = And(x=w501, y=w502) -> (x .and. y?=w497:bool)
                          n423 = Or(x=w498, y=w497) -> (x .or. y?=w496:bool)
                          n424 = Or(x=w496, y=w507) -> (x .or. y?=w508:bool)
                        }
                        n425 = local write "Calculate condition"(TRUE ("Calculate condition")) -> ()
                      }
                      frame #2 {
                        n426 = flat-sequence {
                          tunnel: w511 -> [w513]
                          tunnel: [w513] -> w510
                          tunnel: w510 -> [w516]
                          frame #0 {
                            n427 = local write "Equlibrating Temperature"(TRUE) -> ()
                          }
                          frame #1 {
                            # "Wait 1.5 system volumes"
                            n428 = local read "tau 2"() -> (w519:dbl)
                            n429 = local read "tau 4"() -> (w523:dbl)
                            n430 = local read "tau 3"() -> (w520:dbl)
                            n431 = local read "tau 5"() -> (w525:dbl)
                            n432 = local read "tau 1"() -> (w518:dbl)
                            n433 = Add(x=w518, y=w519) -> (x+y=w521:dbl)
                            n434 = Add(x=w521, y=w520) -> (x+y=w522:dbl)
                            n435 = Add(x=w522, y=w523) -> (x+y=w524:dbl)
                            n436 = Add(x=w524, y=w525) -> (x+y=w526:dbl)
                            "Total System Resisdence Time(min)" <- w526
                            n437 = Multiply(x=w526, y=1.5) -> (x*y=w517:dbl)
                            "total_flush_time(min)" <- w517
                            n438 = Multiply(x=60.0, y=w517) -> (x*y=w514:dbl)
                            n439 = script code="start = tic;\ntotal_wait_time1 = 30;"("total_wait_time"=w514) -> ("??"=w515:errorcluster)  [unwired: 1 in]
                            n440 = property on="System Flush Wait Time" class="Slide (strict)"("Scale.Maximum"=w514) -> ()  [unwired: 2 in, 2 out]
                            n441 = while {
                              tunnel: w516 -> [w533]
                              tunnel: w515 -> [w532]
                              stop <- w534 stop-if-true
                              # "Check if system is flushed every 10 seconds"
                              n442 = script code="end1 = toc(start);\nflush_time = 0;\n\nif end1 > total_wait_time1\n   flush_time = 1;\nend\ncurr_wait_time = end1 /60;"("??"=w532) -> ("flush_time"=w537:dbl, "curr_wait_time"=w531:dbl)  [unwired: 1 out]
                              "curr_wait_time(min)" <- w531
                              n443 = Multiply(x=w531, y=60.0) -> (x*y=w529:dbl)
                              n444 = Not Equal To 0?(x=w537) -> (x != 0?=w536:bool)
                              "System Flushed?" <- w536
                              n445 = local read "Stop"() -> (w539:bool)
                              n446 = local write "System Flush Wait Time"(w529) -> ()
                              n447 = Or(x=w536, y=w539) -> (x .or. y?=w535:bool)
                              n448 = Or(x=w535, y=w533) -> (x .or. y?=w534:bool)
                              n449 = Wait (ms)(milliseconds to wait=u32 500) -> ()  [unwired: 1 out]
                            }
                          }
                        }
                      }
                      frame #3 {
                        # "Collect HPLC Data"
                        n450 = flat-sequence {
                          tunnel: w541 -> [w544]
                          tunnel: [w575] -> w540
                          frame #0 {
                            # "Switch Valve to\n Load position"
                            n451 = local write "Flushing System"(TRUE ("Flushing System")) -> ()
                          }
                          frame #1 {
                            # "Start Method"
                          }
                          frame #2 {
                            # "Fill SL"
                            n452 = Wait (ms)(milliseconds to wait=u32 5000) -> ()  [unwired: 1 out]
                          }
                          frame #3 {
                          }
                          frame #4 {
                            # "Inject \nSample"
                          }
                          frame #5 {
                            # "Reduce pump flowrates during hplc analysis"
                            n453 = stacked-sequence {
                              tunnel: w544 -> [w549 w550 w555 w560 w565 w570]
                              frame #0 {
                                n454 = Index Array(array=w549, index=0) -> (element=w547:dbl)
                                n455 = Greater Than 0?(x=w547) -> (x > 0?=w546:bool)
                                n456 = case shown="False" w546 {
                                tunnel: 10.0 ("Flowrate(ul/min)") -> [_ _]
                                frame False {
                                }
                                frame True {
                                }
                                }
                              }
                              frame #1 {
                                (unwired) 10.0 ("Flowrate(ul/min)")
                                n457 = Index Array(array=w550, index=1) -> (element=w552:dbl)
                                n458 = Greater Than 0?(x=w552) -> (x > 0?=w551:bool)
                                n459 = case shown="True" w551 {
                                frame False {
                                }
                                frame True {
                                n460 = local read "Syringe_pump?"() -> (w554:bool)
                                n461 = case shown="False" w554 {
                                frame False {
                                }
                                frame True {
                                }
                                }
                                }
                                }
                              }
                              frame #2 {
                                n462 = Index Array(array=w555, index=2) -> (element=w558:dbl)
                                n463 = Greater Than 0?(x=w558) -> (x > 0?=w557:bool)
                                n464 = case shown="True" w557 {
                                tunnel: 10.0 ("Flowrate(ul/min)") -> [_ _]
                                frame False {
                                }
                                frame True {
                                }
                                }
                              }
                              frame #3 {
                                n465 = Index Array(array=w560, index=3) -> (element=w563:dbl)
                                n466 = Greater Than 0?(x=w563) -> (x > 0?=w562:bool)
                                n467 = case shown="False" w562 {
                                tunnel: 10.0 ("Flowrate(ul/min)") -> [_ _]
                                frame False {
                                }
                                frame True {
                                }
                                }
                              }
                              frame #4 {
                                n468 = Index Array(array=w565, index=4) -> (element=w568:dbl)
                                n469 = Greater Than 0?(x=w568) -> (x > 0?=w567:bool)
                                n470 = case shown="True" w567 {
                                tunnel: 10.0 ("Flowrate(ul/min)") -> [_ _]
                                frame False {
                                }
                                frame True {
                                }
                                }
                              }
                              frame #5 {
                                n471 = Index Array(array=w570, index=5) -> (element=w573:dbl)
                                n472 = Greater Than 0?(x=w573) -> (x > 0?=w572:bool)
                                n473 = case shown="True" w572 {
                                tunnel: 10.0 ("Flowrate(ul/min)") -> [_ _]
                                frame False {
                                }
                                frame True {
                                }
                                }
                              }
                            }
                          }
                          frame #6 {
                            # "Analyze Peaks"
                            n474 = local read "Bay Parameters"() -> (w576:T4)
                            n475 = Unbundle By Name(w576) -> ("HPLC File Name"=w577:string)
                            n476 = disable-structure shown="Disabled" {
                              disable-tunnel: w577 -> [w580 _]
                              frame Disabled {
                                n477 = call "hplc_analyze.vi"("File Path"=w580) -> ()  [unwired: 10 in, 1 out]
                              }
                              frame Enabled {
                              }
                            }
                            n478 = flat-sequence {
                              tunnel: w576 -> [w579]
                              tunnel: [w579] -> w575
                              frame #0 {
                                n479 = One Button Dialog(message="Click Ok") -> ()  [unwired: 1 in, 1 out]
                              }
                            }
                          }
                        }
                      }
                      frame #4 {
                        # "Save data to excel file"
                        n480 = script code="if not(system_error) && not(redo)\n  if opt_ctr == 1\n     if total_wait_time < 7.5*60\n        f(req_ctr,:) = [-(C_measured) sqrt(eps)];  \n     else\n         f(req_ctr,:) = [0 sqrt(eps)];\n     end \n     %f(req_ctr,:) = [-C_measured/total_wait_time sqrt(eps)];  \n  end\n  temp_write = [CurrExp, f(req_ctr,1), C_measured];\n  lastrowStr4 = num2str(lastrow4);\n  xlSheets.Item(idx4).Range(strcat('A',lastrowStr4,':',lastcol4,lastrowStr4)).Value2 =  temp_write;\n  lastrow4 = lastrow4 +1;\n  xlWorkbook.SaveAs(xl_file);\n  allHPLCData(end+1,:) =  [CurrExp new_x(:)' f(req_ctr,1) C_measured]\n  %allHPLCFile(end+1,:) = [num2str(CurrExp) hplc_file];\n\n  opt_ctr = 1;\n  CurrExp = CurrExp + 1;\n  terminate = 0;\n\n    if is_first_set_of_exp\n       ncall0 = size(f,1);\n       is_first_set_of_exp = false;\n    else\n       ncall0 = ncall0 +1;% size(f,1); % update function call counter\n    end\n    [fbestn,jbest] = min(f(:,1)); % best function value\n\n    if fbestn < fbest\n        fbest = fbestn;\n        xbest = x(jbest,:);\n        ncall0,xbest,fbest % display current number of function values,\n        % best point and function value if fbest has changed\n        nstop0 = 0;\n   \n    end\n  \n      % check stopping criterion\n    if nstop0 >= nstop  || ncall0 >= ncall\n       terminate = 1;\n       lastrowStr_temp = num2str(10);\n       lastcol_temp =  xlcolumnletter(length(xbest)+1);\n       xlSheets.Item(idx3).Range(strcat('B',lastrowStr_temp,':',lastcol_temp,lastrowStr_temp)).Value2 =  xbest;\n       xlWorkbook.SaveAs(xl_file);\n    end\n\n    if req_ctr == req_tot\n        if ncall >= minfcall && fbestn > fbest\n           nstop0 = nstop0 + 1;\n        end\n       opt_ctr = 3;\n    else\n       req_ctr = req_ctr +1;\n    end\n\n   save(matlabsavefile);\nend  \n \n  %Conc = reactor_obj_fun(params_1);\n  %temp_write = [CurrExp, Conc];\n  %lastrowStr4 = num2str(lastrow4);\n  %xlSheets.Item(idx4).Range(strcat('A',lastrowStr4,':',lastcol4,lastrowStr4)).Value2 =  temp_write;\n  %lastrow4 = lastrow4 +1;\n  %xlWorkbook.SaveAs(xl_file);\n\n  %f(req_ctr,:) = [Conc sqrt(eps)];\n  %opt_ctr = 1;\n  %CurrExp = CurrExp + 1;\n  %terminate = 0;\n\n\n    %if is_first_set_of_exp\n     %  ncall0 = size(f,1);\n      % is_first_set_of_exp = false;\n    %else\n       %ncall0 = ncall0 +1;% size(f,1); % update function call counter\n    %end\n    %[fbestn,jbest] = min(f(:,1)); % best function value\n\n    %if fbestn < fbest\n     %   fbest = fbestn;\n     %   xbest = x(jbest,:);\n     %   ncall0,xbest,fbest % display current number of function values,\n     %   % best point and function value if fbest has changed\n     %   nstop0 = 0;\n   \n   % end\n  \n      % check stopping criterion\n    %if nstop0 >= nstop  || ncall0 >= ncall\n    %   terminate = 1;\n     %  lastrowStr_temp = num2str(10);\n     %  lastcol_temp =  xlcolumnletter(length(xbest)+1);\n     %  xlSheets.Item(idx3).Range(strcat('B',lastrowStr_temp,':',lastcol_temp,lastrowStr_temp)).Value2 =  xbest;\n     %  xlWorkbook.SaveAs(xl_file);\n   % end\n\n    %if req_ctr == req_tot\n    %    if ncall >= minfcall && fbestn > fbest\n    %       nstop0 = nstop0 + 1;\n    %    end\n    %   opt_ctr = 3;\n   % else\n    %   req_ctr = req_ctr +1;\n   % end\n\n   %save(matlabsavefile);"() -> ("terminate"=w581:dbl)  [unwired: 1 in, 1 out]
                      }
                      frame #5 {
                        n481 = local read "Num_exp_till_pause"() -> (w584:i32)
                        n482 = Increment(x=w584) -> (x+1=w583:i32)
                        n483 = local write "Num_exp_till_pause"(w583) -> ()
                        n484 = local write "HPLC Analysis"(TRUE ("HPLC Analysis")) -> ()
                      }
                      frame #6 {
                        # "Pause System"
                        n485 = local read "Bay Parameters"() -> (w592:T4)
                        n486 = Unbundle By Name(w592) -> ("Num_conditons_per_wait"=w591:dbl)
                        n487 = local read "Num_exp_till_pause"() -> (w590:i32)
                        n488 = Equal?(x=w591, y=w590) -> (x = y?=w589:bool)
                        n489 = local read "Run_Stop_cluster"() -> (w586:T6)
                        n490 = Unbundle By Name(w586) -> ("Stop Run Button"=w588:bool)
                        n491 = Or(x=w588, y=w589) -> (x .or. y?=w587:bool)
                        n492 = case shown="False" w587 {
                          tunnel: w591 -> [w595 _]
                          tunnel: w590 -> [w596 _]
                          tunnel: w586 -> [_ w598]
                          frame False {
                            n493 = Greater?(x=w596, y=w595) -> (0:w594:bool)
                            n494 = case shown="False" w594 {
                              frame False {
                              }
                              frame True {
                                n495 = local write "Num_exp_till_pause"(0 ("Num_exp_till_pause")) -> ()
                              }
                            }
                          }
                          frame True {
                            n496 = flat-sequence {
                              tunnel: w598 -> [w620]
                              frame #0 {
                                w602 = string[] ["e", "f", "g", "h", "i", "j"]
                                # "Turn off pumps and stop controling temperature"
                                n497 = stacked-sequence {
                                frame #0 {
                                n498 = local write "Temperature Control 1"(FALSE ("Temperature Control 1")) -> ()
                                }
                                frame #1 {
                                n499 = local write "Temperature Control 2"(FALSE ("Temperature Control 2")) -> ()
                                }
                                frame #2 {
                                n500 = local write "Temperature Control 3"(FALSE ("Temperature Control 3")) -> ()
                                }
                                frame #3 {
                                n501 = local write "Temperature Control 4"(FALSE ("Temperature Control 4")) -> ()
                                }
                                frame #4 {
                                n502 = local write "Temperature Control 5"(FALSE ("Temperature Control 5")) -> ()
                                }
                                }
                                n503 = local read "COMM Port:: Harvard Syringe Pump"() -> (w600:refnum<visa-resource-name>)
                                n504 = local read "Syringe_pump?"() -> (w599:bool)
                                n505 = local read "COMM Port :: Milligat Pumps"() -> (w601:refnum<visa-resource-name>)
                                n506 = Array Size(array=w602) -> (size(s)=w603:i32)
                                n507 = case shown="True" w599 {
                                tunnel: w600 -> [_ _]
                                frame False {
                                }
                                frame True {
                                }
                                }
                                n508 = for {
                                N: w603 -> [_]
                                tunnel: w602 -> [_] mode=indexing
                                tunnel: w601 -> [_]
                                }
                              }
                              frame #1 {
                                n509 = while {
                                stop <- w614 stop-if-true
                                # "Wait till user confirms system resume"
                                n510 = Two Button Dialog(message="System is currently paused. Refill Syringes, flush lines, then press OK to continue optimization.\nOr Redo to repeat condition ", 1:"REDO" ("F button name (\"Cancel\")"), 2:"OK" ("Left Button Text (\"Yes\")")) -> (T button?=w610:bool)
                                n511 = local read "Stop"() -> (w615:bool)
                                n512 = case shown="False" w610 {
                                tunnel: [TRUE TRUE] -> w609
                                frame False {
                                n513 = script code="redo = true;"() -> ()  [unwired: 1 in, 1 out]
                                }
                                frame True {
                                }
                                }
                                n514 = Or(x=w609, y=w615) -> (x .or. y?=w614:bool)
                                }
                              }
                              frame #2 {
                                n515 = local write "Num_exp_till_pause"(0 ("Num_exp_till_pause")) -> ()
                                n516 = Bundle By Name(cluster=w620, "Stop Run Button"=FALSE) -> (w618:T6)
                                n517 = local write "Run_Stop_cluster"(w618) -> ()
                              }
                            }
                          }
                        }
                      }
                      frame #7 {
                        w623 = FALSE
                        n518 = local write "Equlibrating Temperature"(w623) -> ()
                        n519 = local write "Calculate condition"(w623) -> ()
                        n520 = local write "Flushing System"(w623) -> ()
                        n521 = local write "HPLC Analysis"(w623) -> ()
                        n522 = local write "stop_xl_write"(TRUE ("stop_xl_write")) -> ()
                      }
                    }
                    n523 = while {
                      stop <- w400 stop-if-true
                      n524 = flat-sequence {
                        frame #0 {
                          n525 = script code="if record_data\n   temp2 = [CurrExp, rem(now,1), P1, P2, P3, P4, P5,P6, T1, T2, T3, T4, T5, T1_SP, T2_SP, T3_SP, T4_SP, T5_SP, F1, F2, Pres1, Pres2];\n   lastrowStr1 = num2str(lastrow1);\n   xlSheets.Item(idx1).Range(strcat('A',lastrowStr1,':',lastcol1,lastrowStr1)).Value2 =  temp2;\n   lastrow1 = lastrow1+1;\n   record_data = false;\nelse\n   record_data = true;\nend"() -> ()  [unwired: 1 in, 1 out]
                        }
                        frame #1 {
                          n526 = Wait (ms)(milliseconds to wait=u32 3000) -> ()  [unwired: 1 out]
                        }
                      }
                      n527 = local read "Stop"() -> (w401:bool)
                      n528 = local read "stop_xl_write"() -> (w402:bool)
                      n529 = Or(x=w402, y=w401) -> (x .or. y?=w400:bool)
                    }
                  }
                  frame True {
                    # "STANDBY MODE"
                    n530 = case shown="False" "Bay Heating 1" {
                      tunnel: [0 1] -> _
                      frame False {
                      }
                      frame True {
                      }
                    }
                    n531 = local read "COMM Port :: Milligat Pumps"() -> (w689:refnum<visa-resource-name>)
                    n532 = case shown="False" "Pump 1" {
                      tunnel: w689 -> [_ _]
                      frame False {
                      }
                      frame True {
                      }
                    }
                    n533 = case shown="False" "Bay Heating 2" {
                      tunnel: [0 1] -> _
                      frame False {
                      }
                      frame True {
                      }
                    }
                    n534 = local read "COMM Port :: Milligat Pumps"() -> (w687:refnum<visa-resource-name>)
                    n535 = case shown="True" "Pump 2" {
                      tunnel: w687 -> [_ _]
                      frame False {
                      }
                      frame True {
                      }
                    }
                    n536 = Add(x=w693, y=2.0) -> (x+y=w695:dbl)
                    n537 = case shown="True" "Bay Heating 3" {
                      tunnel: [0 1] -> _
                      frame False {
                      }
                      frame True {
                      }
                    }
                    n538 = local read "COMM Port :: Milligat Pumps"() -> (w685:refnum<visa-resource-name>)
                    n539 = case shown="True" "Pump 3" {
                      tunnel: w685 -> [_ _]
                      frame False {
                      }
                      frame True {
                      }
                    }
                    n540 = Wait (ms)(milliseconds to wait=u32 1000) -> ()  [unwired: 1 out]
                    n541 = case shown="True" "Bay Heating 4" {
                      tunnel: [0 1] -> _
                      frame False {
                      }
                      frame True {
                      }
                    }
                    n542 = local read "COMM Port :: Milligat Pumps"() -> (w683:refnum<visa-resource-name>)
                    n543 = case shown="True" "Pump 4" {
                      tunnel: w683 -> [_ _]
                      frame False {
                      }
                      frame True {
                      }
                    }
                    n544 = case shown="True" "Bay Heating 5" {
                      tunnel: [0 1] -> _
                      frame False {
                      }
                      frame True {
                      }
                    }
                    n545 = local read "COMM Port :: Milligat Pumps"() -> (w681:refnum<visa-resource-name>)
                    n546 = case shown="True" "Pump 5" {
                      tunnel: w681 -> [_ _]
                      frame False {
                      }
                      frame True {
                      }
                    }
                    n547 = local read "COMM Port :: Milligat Pumps"() -> (w679:refnum<visa-resource-name>)
                    n548 = case shown="True" "Pump 6" {
                      tunnel: w679 -> [_ _]
                      frame False {
                      }
                      frame True {
                      }
                    }
                  }
                }
                n549 = Less?(x=w374, y=w377) -> (x < y?=w375:bool)
                n550 = Equal?(x=w372, y=1.0) -> (x = y?=w369:bool)
                n551 = local read "Stop"() -> (w376:bool)
                n552 = Or(x=w376, y=w375) -> (x .or. y?=w371:bool)
                n553 = Or(x=w369, y=w371) -> (x .or. y?=w370:bool)
                n554 = case shown="True" w369 {
                  frame False {
                  }
                  frame True {
                    n555 = local write "Stop"(TRUE ("Stop")) -> ()
                  }
                }
                "Optimization_loop_index" <- w378
              }
            }
          }
          n556 = while {
            stop <- w769 stop-if-true
            n557 = local read "Temperature Control 3"() -> (w765:bool)
            n558 = local read "Debug_run_button"() -> (w766:bool)
            n559 = Not(x=w766) -> (.not. x?=w768:bool)
            n560 = And(x=w768, y=w765) -> (x .and. y?=w767:bool)
            n561 = case shown="True" w767 {
              frame False {
                n562 = local write "Temp SS? 3"(TRUE) -> ()
              }
              frame True {
                # "Bay 3 Temperature Controller"
                n563 = local read "Temperature SP 3"() -> (w772:dbl)
                n564 = local read "Temperature 3"() -> (w773:dbl)
                n565 = Subtract(x=w773, y=w772) -> (x-y=w775:dbl)
                n566 = Absolute Value(x=w775) -> (abs(x)=w777:dbl)
                n567 = Less Or Equal?(x=w777, y=1.2) -> (x <= y?=w774:bool)
                n568 = local write "Temp SS? 3"(w774) -> ()
                n569 = local read "SSR Duration 3"() -> (w785:dbl)
                n570 = call-poly <vilib>:"PID Online Autotuning.vi"("setpoint"=w772, "manipulated variable"=w785, "autotuning parameters"=T8 {"type of controller"=enum."PID", "relay cycles"=3, "relay amplitude"=1.0, "control specifications"=enum."Normal", "PV noise level"=0.1} ("Autotuning Parameters R1"), "process variable"=w773, "PID gains in"=T7 {"Proportional gain Kc"=0.38538, "Integral time Ti (sec)"=0.524375, "Derivative time Ti (sec)"=0.12585} ("PID gains 2")) -> ("setpoint out"=w783:dbl, "process variable out"=w784:dbl, "PID gains out"=w787:T9)  [unwired: 6 in, 2 out]
                n571 = call <vilib>:"PID Autotuning (Temperature).vi"("desired temperature"=w783, "measured temperature"=w784, "PID gains in"=w787, "output range"=cluster{"output high":dbl, "output low":dbl} {"output high"=3.0, "output low"=-1.0} ("Output range")) -> ("output"=w779:dbl)  [unwired: 12 in, 3 out]
                n572 = Multiply(x=1000.0, y=w779) -> (x*y=w781:dbl)
                n573 = local write "SSR Duration 3"(w779) -> ()
                n574 = Greater Than 0?(x=w781) -> (x > 0?=w782:bool)
                n575 = case shown="False" w782 {
                  tunnel: 4 -> [_ _]
                  tunnel: w781 -> [w790 _]
                  frame False {
                    (unwired) errorcluster {"status"=FALSE, "code"=0, "source"=""} ("error out")
                    n576 = Absolute Value(x=w790) -> (abs(x)=w791:dbl)
                    n577 = Wait (ms)(milliseconds to wait=w791) -> ()  [unwired: 1 out]
                  }
                  frame True {
                  }
                }
              }
            }
            n578 = Wait (ms)(milliseconds to wait=u32 300) -> ()  [unwired: 1 out]
            n579 = local read "Stop"() -> (w769:bool)
          }
          n580 = while {
            stop <- w742 stop-if-true
            n581 = local read "Debug_run_button"() -> (w738:bool)
            n582 = Not(x=w738) -> (.not. x?=w741:bool)
            n583 = Wait (ms)(milliseconds to wait=u32 300) -> ()  [unwired: 1 out]
            n584 = local read "Temperature Control 4"() -> (w740:bool)
            n585 = And(x=w741, y=w740) -> (x .and. y?=w739:bool)
            n586 = case shown="True" w739 {
              frame False {
                n587 = local write "Temp SS? 4"(TRUE ("Temp SS? 4")) -> ()
              }
              frame True {
                # "Bay 4 Temperature Controller"
                n588 = local read "Temperature SP 4"() -> (w745:dbl)
                n589 = local read "Temperature 4"() -> (w746:dbl)
                n590 = Subtract(x=w746, y=w745) -> (x-y=w748:dbl)
                n591 = Absolute Value(x=w748) -> (abs(x)=w750:dbl)
                n592 = Less Or Equal?(x=w750, y=1.2) -> (x <= y?=w747:bool)
                n593 = local write "Temp SS? 4"(w747) -> ()
                n594 = local read "SSR Duration 4"() -> (w751:dbl)
                n595 = call-poly <vilib>:"PID Online Autotuning.vi"("setpoint"=w745, "manipulated variable"=w751, "autotuning parameters"=T8 {"type of controller"=enum."PID", "relay cycles"=3, "relay amplitude"=1.0, "control specifications"=enum."Normal", "PV noise level"=0.1} ("Autotuning Parameters R1"), "process variable"=w746, "PID gains in"=T7 {"Proportional gain Kc"=0.38538, "Integral time Ti (sec)"=0.524375, "Derivative time Ti (sec)"=0.12585} ("PID gains 2")) -> ("setpoint out"=w753:dbl, "process variable out"=w754:dbl, "PID gains out"=w756:T9)  [unwired: 6 in, 2 out]
                n596 = call <vilib>:"PID Autotuning (Temperature).vi"("desired temperature"=w753, "measured temperature"=w754, "PID gains in"=w756, "output range"=cluster{"output high":dbl, "output low":dbl} {"output high"=3.0, "output low"=-1.0} ("Output range")) -> ("output"=w752:dbl)  [unwired: 12 in, 3 out]
                n597 = Multiply(x=1000.0, y=w752) -> (x*y=w760:dbl)
                n598 = Greater Than 0?(x=w760) -> (x > 0?=w761:bool)
                n599 = local write "SSR Duration 4"(w752) -> ()
                n600 = case shown="False" w761 {
                  tunnel: 5 -> [_ _]
                  tunnel: w760 -> [w763 _]
                  frame False {
                    (unwired) errorcluster {"status"=FALSE, "code"=0, "source"=""} ("error out")
                    n601 = Absolute Value(x=w763) -> (abs(x)=w764:dbl)
                    n602 = Wait (ms)(milliseconds to wait=w764) -> ()  [unwired: 1 out]
                  }
                  frame True {
                  }
                }
              }
            }
            n603 = local read "Stop"() -> (w742:bool)
          }
          n604 = while {
            stop <- w715 stop-if-true
            n605 = local read "Debug_run_button"() -> (w712:bool)
            n606 = Not(x=w712) -> (.not. x?=w714:bool)
            n607 = local read "Temperature Control 5"() -> (w711:bool)
            n608 = And(x=w714, y=w711) -> (x .and. y?=w713:bool)
            n609 = case shown="True" w713 {
              frame False {
                n610 = local write "Temp SS? 5"(TRUE ("Temp SS? 5")) -> ()
              }
              frame True {
                # "Bay 5 Temperature Controller"
                n611 = local read "SSR Duration 5"() -> (w724:dbl)
                n612 = local read "Temperature SP 5"() -> (w718:dbl)
                n613 = local read "Temperature 5"() -> (w719:dbl)
                n614 = Subtract(x=w719, y=w718) -> (x-y=w721:dbl)
                n615 = Absolute Value(x=w721) -> (abs(x)=w723:dbl)
                n616 = Less Or Equal?(x=w723, y=1.2) -> (x <= y?=w720:bool)
                n617 = local write "Temp SS? 5"(w720) -> ()
                n618 = call-poly <vilib>:"PID Online Autotuning.vi"("setpoint"=w718, "manipulated variable"=w724, "autotuning parameters"=T8 {"type of controller"=enum."PID", "relay cycles"=3, "relay amplitude"=1.0, "control specifications"=enum."Normal", "PV noise level"=0.1} ("Autotuning Parameters R1"), "process variable"=w719, "PID gains in"=T7 {"Proportional gain Kc"=0.38538, "Integral time Ti (sec)"=0.524375, "Derivative time Ti (sec)"=0.12585} ("PID gains 2")) -> ("setpoint out"=w726:dbl, "process variable out"=w727:dbl, "PID gains out"=w729:T9)  [unwired: 6 in, 2 out]
                n619 = call <vilib>:"PID Autotuning (Temperature).vi"("desired temperature"=w726, "measured temperature"=w727, "PID gains in"=w729, "output range"=cluster{"output high":dbl, "output low":dbl} {"output high"=3.0, "output low"=-1.0} ("Output range")) -> ("output"=w725:dbl)  [unwired: 12 in, 3 out]
                n620 = Multiply(x=1000.0, y=w725) -> (x*y=w733:dbl)
                n621 = Greater Than 0?(x=w733) -> (x > 0?=w734:bool)
                n622 = local write "SSR Duration 5"(w725) -> ()
                n623 = case shown="False" w734 {
                  tunnel: 6 -> [_ _]
                  tunnel: w733 -> [w736 _]
                  frame False {
                    (unwired) errorcluster {"status"=FALSE, "code"=0, "source"=""} ("error out")
                    n624 = Absolute Value(x=w736) -> (abs(x)=w737:dbl)
                    n625 = Wait (ms)(milliseconds to wait=w737) -> ()  [unwired: 1 out]
                  }
                  frame True {
                  }
                }
              }
            }
            n626 = Wait (ms)(milliseconds to wait=u32 300) -> ()  [unwired: 1 out]
            n627 = local read "Stop"() -> (w715:bool)
          }
        }
      }
      n628 = while {
        tunnel: errorcluster {"status"=FALSE, "code"=0, "source"=""} ("error out") -> [w113]
        stop <- w132 stop-if-true
        # "Bay 5 Temperature Read"
        # "Bay 4 Temperature Read"
        # "Bay 3 Temperature Read"
        # "Bay 2 Temperature Read"
        # "Bay 1 Temperature Read"
        n629 = local read "Temperature SP 1"() -> (w115:dbl)
        n630 = local read "Stop"() -> (w132:bool)
        n631 = local write "error out"(w113) -> ()
        n632 = Unbundle By Name(w113) -> ("status"=w129:bool)
        n633 = call-poly <vilib>:"PID Control Input Filter.vi"("input"=w115) -> ("output"=w127:dbl)  [unwired: 4 in]
        n634 = case shown="False" w129 {
          tunnel: w127 -> [w141 _]
          tunnel: [w141 w142] -> w128
          frame False {
            n635 = local write "Temperature 1"(w141) -> ()
          }
          frame True {
            n636 = local read "Temperature 1"() -> (w142:dbl)
          }
        }
        n637 = flat-sequence {
          frame #0 {
            n638 = Wait (ms)(milliseconds to wait=u32 500) -> ()  [unwired: 1 out]
          }
        }
        n639 = local read "Temperature SP 2"() -> (w114:dbl)
        n640 = Unbundle By Name(w113) -> ("status"=w126:bool)
        n641 = local write "error out"(w113) -> ()
        n642 = call-poly <vilib>:"PID Control Input Filter.vi"("input"=w114) -> ("output"=w125:dbl)  [unwired: 4 in]
        n643 = case shown="True" w126 {
          tunnel: w125 -> [w139 _]
          tunnel: [w139 w140] -> w124
          frame False {
            n644 = local write "Temperature 2"(w139) -> ()
          }
          frame True {
            n645 = local read "Temperature 2"() -> (w140:dbl)
          }
        }
        n646 = local read "Temperature SP 3"() -> (w110:dbl)
        n647 = local write "error out"(w113) -> ()
        n648 = Unbundle By Name(w113) -> ("status"=w121:bool)
        n649 = call-poly <vilib>:"PID Control Input Filter.vi"("input"=w110) -> ("output"=w123:dbl)  [unwired: 4 in]
        n650 = case shown="True" w121 {
          tunnel: w123 -> [w137 _]
          tunnel: [w137 w138] -> w122
          frame False {
            n651 = local write "Temperature 3"(w137) -> ()
          }
          frame True {
            n652 = local read "Temperature 3"() -> (w138:dbl)
          }
        }
        n653 = local write "error out"(w113) -> ()
        n654 = Unbundle By Name(w113) -> ("status"=w118:bool)
        n655 = local read "Temperature SP 4"() -> (w111:dbl)
        n656 = local read "Temperature SP 5"() -> (w112:dbl)
        n657 = call-poly <vilib>:"PID Control Input Filter.vi"("input"=w111) -> ("output"=w120:dbl)  [unwired: 4 in]
        n658 = case shown="True" w118 {
          tunnel: w120 -> [w135 _]
          tunnel: [w135 w136] -> w119
          frame False {
            n659 = local write "Temperature 4"(w135) -> ()
          }
          frame True {
            n660 = local read "Temperature 4"() -> (w136:dbl)
          }
        }
        n661 = local write "error out"(w113) -> ()
        n662 = Unbundle By Name(w113) -> ("status"=w116:bool)
        n663 = Build Array(w128, w124, w122, w119, w112) -> (w131:dbl[])
        n664 = Array To Cluster(array=w131) -> (cluster=→"Teperature Chart":T5)
        n665 = case shown="False" w116 {
          tunnel: w112 -> [w133 _]
          tunnel: [w133 w134] -> w117
          frame False {
            n666 = local write "Temperature 5"(w133) -> ()
          }
          frame True {
            n667 = local read "Temperature 5"() -> (w134:dbl)
          }
        }
        n668 = script code="MATLAB script"("T1"=w128, "T2"=w124, "T3"=w122, "T4"=w119, "T5"=w117) -> ()  [unwired: 1 in, 1 out]
      }
      n669 = disable-structure shown="Disabled" {
        frame Disabled {
          n670 = while {
            stop <- w46 stop-if-true
            # "Collect MS Data"
            n671 = local read "MS task"() -> (w44:refnum<k21>)
            n672 = call-poly <vilib>:"DAQmx Read.vi"("task/channels in"=w44) -> ("data"=w43:dbl[])  [unwired: 12 in, 2 out]
            "MS Array" <- w43
            n673 = script code="MATLAB script"("MS_Data"=w43) -> ()  [unwired: 1 in, 1 out]
            n674 = Build Array(w43) -> (→"MS Signals Chart":dbl[][])
            n675 = local read "Stop"() -> (w46:bool)
            n676 = Wait (ms)(milliseconds to wait=u32 300) -> ()  [unwired: 1 out]
          }
        }
        frame Enabled {
        }
      }
      n677 = while {
        stop <- w53 stop-if-true
        n678 = local read "Pump setpoint(ul/min) 1"() -> (w56:dbl)
        n679 = local read "Pump setpoint(ul/min) 2"() -> (w52:dbl)
        n680 = local read "Pump setpoint(ul/min) 3"() -> (w51:dbl)
        n681 = local read "Pump setpoint(ul/min) 4"() -> (w50:dbl)
        n682 = local read "Pump setpoint(ul/min) 5"() -> (w49:dbl)
        n683 = local read "Pump setpoint(ul/min) 6"() -> (w48:dbl)
        n684 = Build Array(w56, w52, w51, w50, w49, w48) -> (w57:dbl[])
        n685 = Array To Cluster(array=w57) -> (cluster=→"Pump Setpoints Chart":T5)
        n686 = Wait (ms)(milliseconds to wait=u32 5000) -> ()  [unwired: 1 out]
        n687 = local read "Stop"() -> (w53:bool)
      }
      n688 = while {
        stop <- w105 stop-if-true
        w58 = dbl[] [1.12, 1.2, 1.0, 0.87]
        w63 = 200
        w74 = 600
        w83 = 600
        # "Read Pressure and Flowrate"
        n689 = local read "Stop"() -> (w105:bool)
        n690 = Index Array(array=w58, index=3) -> (element=w97:dbl)
        n691 = Index Array(array=w58, index=2) -> (element=w98:dbl)
        n692 = Index Array(array=w58, index=1) -> (element=w99:dbl)
        n693 = Index Array(array=w58, index=0) -> (element=w100:dbl)
        n694 = call-poly <vilib>:"PID Control Input Filter.vi"("input"=w97) -> ("output"=w90:dbl)  [unwired: 4 in]
        n695 = call-poly <vilib>:"PID Control Input Filter.vi"("input"=w98) -> ("output"=w89:dbl)  [unwired: 4 in]
        n696 = call-poly <vilib>:"PID Control Input Filter.vi"("input"=w100) -> ("output"=w79:dbl)  [unwired: 4 in]
        n697 = call-poly <vilib>:"PID Control Input Filter.vi"("input"=w99) -> ("output"=w70:dbl)  [unwired: 4 in]
        n698 = Subtract(x=w79, y=0.065) -> (x-y=w80:dbl)
        n699 = Subtract(x=w70, y=0.065) -> (x-y=w71:dbl)
        n700 = Multiply(x=104.96 ("y"), y=w90) -> (x*y=w91:dbl)
        n701 = Multiply(x=104.96 ("y"), y=w89) -> (x*y=w94:dbl)
        n702 = Subtract(x=w91, y=24.077) -> (x-y=w61:dbl)
        n703 = Multiply(x=2, y=w83) -> (x*y=w85:i32)
        n704 = Divide(x=w85, y=3.3) -> (x/y=w81:dbl)
        n705 = Multiply(x=w80, y=w81) -> (x*y=w82:dbl)
        n706 = Subtract(x=w82, y=w83) -> (x-y=w65:dbl)
        n707 = Subtract(x=w94, y=24.077) -> (x-y=w62:dbl)
        n708 = Multiply(x=2, y=w74) -> (x*y=w76:i32)
        n709 = Divide(x=w76, y=3.3) -> (x/y=w72:dbl)
        n710 = Multiply(x=w71, y=w72) -> (x*y=w73:dbl)
        n711 = Subtract(x=w73, y=w74) -> (x-y=w64:dbl)
        n712 = Build Array(w65, w64) -> (w68:dbl[])
        n713 = Array To Cluster(array=w68) -> (cluster=→"Flowrate Chart":T5)
        n714 = Build Array(w62, w61) -> (w69:dbl[])
        n715 = local write "Flowrate Sensor 1"(w65) -> ()
        n716 = local write "Flowrate Sensor 2"(w64) -> ()
        n717 = local write "Pressure 1"(w62) -> ()
        n718 = local write "Pressure 2"(w61) -> ()
        n719 = Array To Cluster(array=w69) -> (cluster=→"Pressure Chart":T5)
        n720 = Wait (ms)(milliseconds to wait=u32 500) -> ()  [unwired: 1 out]
        n721 = script code="MATLAB script"("F1"=w65, "F2"=w64, "Pres1"=w62, "Pres2"=w61) -> ()  [unwired: 1 in, 1 out]
        n722 = Greater?(x=w61, y=w63) -> (0:w59:bool)
        n723 = Greater?(x=w62, y=w63) -> (0:w60:bool)
        n724 = case shown="True" w60 {
          frame False {
          }
          frame True {
            w109 = TRUE ("Stop")
            n725 = local write "System Error"(w109) -> ()
            n726 = local write "Stop"(w109) -> ()
            n727 = local write "Error Message"("Pressure Sensor 1 readings above 200psi") -> ()
          }
        }
        n728 = case shown="True" w59 {
          frame False {
          }
          frame True {
            w107 = TRUE ("Stop")
            n729 = local write "System Error"(w107) -> ()
            n730 = local write "Stop"(w107) -> ()
            n731 = local write "Error Message"("Pressure Sensor 2 readings above 200psi") -> ()
          }
        }
      }
    }
    frame #3 {
      # "Save and close xml and excel file"
      n732 = script code="if exist('xl_file','var') & exist('xlApp','var')\n  xlWorkbook.SaveAs(xl_file);\n  xlWorkbook.Close;\n  xlApp.Quit;\n  xlApp.delete;\nend"() -> ()  [unwired: 1 in, 1 out]
    }
    frame #4 {
      w853 = string[] ["e", "f", "g", "h", "i", "j"]
      # "End communication to hardware"
      n733 = local read "Syringe_pump?"() -> (w851:bool)
      n734 = local read "COMM Port:: Harvard Syringe Pump"() -> (w852:refnum<visa-resource-name>)
      n735 = local read "COMM Port :: Milligat Pumps"() -> (w855:refnum<visa-resource-name>)
      n736 = Array Size(array=w853) -> (size(s)=w854:i32)
      n737 = case shown="False" w851 {
        tunnel: w852 -> [_ _]
        frame False {
        }
        frame True {
        }
      }
      n738 = for {
        N: w854 -> [_]
        tunnel: w853 -> [_] mode=indexing
        tunnel: w855 -> [_]
      }
    }
    frame #5 {
      # "Display Error Messages if necessary"
      n739 = local read "Error Message"() -> (w857:string)
      n740 = String Length(string=w857) -> (length=w858:i32)
      n741 = Greater Than 0?(x=w858) -> (x > 0?=w856:bool)
      n742 = case shown="True" w856 {
        tunnel: w857 -> [_ w859]
        frame False {
        }
        frame True {
          n743 = One Button Dialog(message=w859) -> ()  [unwired: 1 in, 1 out]
        }
      }
    }
  }
